vi "TLB Native Dynamic Events ver 0.13f.vi"() -> ()   [LabVIEW 2018]
uses:
  Labview Training Phase 2/Enum Controls/States for Action Engine.ctl
  TLB Type Definitions/State Type Definitions, for 0.26d versions and later.ctl
  TLB Type Definitions/Intruction Type Definitions.ctl
  TLB Type Definitions/Encoder cluster.ctl
  TLB Type Definitions/PING CLUSTER.ctl
  <vilib>/Studica/Studica Toolkit/NavX/NavX.lvlib
  <vilib>/Studica/Studica Toolkit/Background/DIO Channel.ctl
  Underlying VI's/NavX VI/navX type def.ctl
  <vilib>/myRIO/Instrument Drivers/Utilities/Utilities.lvlib
  <vilib>/Studica/Studica Toolkit/Background/I2C Channel.ctl
  TLB Type Definitions/Vision cluster.ctl
  <vilib>/NI_Real-Time Target Support.lvlib
  TLB Type Definitions/Stepper cluster.ctl
  Experimental VI's/Archived VI's/MOTOR CONTROL NO PID Type Def.ctl
  Underlying VI's/I2C Master VI/I2C MASTER Type Def.ctl
  Underlying VI's/I2C Master VI/I2C_MASTER_WRITE_NEW Type Def.ctl
  Underlying VI's/Webcam FGV Low level ver/State control.ctl
  <vilib>/userdefined/High Color/IMAQdx.ctl
  Underlying VI's/I2C Master VI/Arduino_Interfacing.ctl
  TLB Type Definitions/Yaw Cluster.ctl
  Experimental VI's/Archived VI's/MOTOR CONTROL NO PID AE DATA ENTRY MODE Type def.ctl
  Experimental VI's/Archived VI's/MOTOR CONTROL NO PID AE DIRECTIONS type def.ctl
  Underlying VI's/Elasped Timer/Control.ctl
  TLB Type Definitions/Time cluster.ctl
  TLB Type Definitions/Y Stepper cluster.ctl
  <vilib>/Utility/RT CPU Load.ctl
panel:
  out "Time up flag":bool
  out "Recognized object + Time up?":bool
  out "Speed & distance":T1
  out "Task selection":u8
  out "Object Center Coordinates":cluster{"x":sgl, "y":sgl}
  out "Object detection cluster":T2
  in  "Object recognition mode":enum16{"Ball", "Soap", "Gel", "Pipe", "None"}(ring)
  out "NavX Readings":T3
  out "Arduino Data":T4
  out "CPU loads":T5[](array[typedef]) {"ISR (%)" format="%#.2f"; "Idle (%)" format="%#.2f"; "Background (%)" format="%#.2f"; "Normal (%)" format="%#.2f"; "Above Normal (%)" format="%#.2f"; "High (%)" format="%#.2g"; "Timed Structures (%)" format="%#.2g"; "Time Critical (%)" format="%#.2g"; "Total (%)" format="%#.2g"}
  in  "Red LED":bool
  out "Detect?":bool
  out "TASK ENABLE":bool
  out "Rising Edge":bool
  in  "Green LED":bool
  out "Object detected?":bool
  out "I2C Error":errorcluster
  out "State Logic":T6=enum."Startup"
  out "elements":T7[](array[typedef])
  in  "STOP TASK":bool
  in  "OK Button":bool
  in  "STOP":bool
  out "error out":errorcluster
  out "Action Queue Items":i32
  out "State Logic Queue Items":i32
  out "Action Queues items":string[](array[string])=["Hardware reset", "Software reset", ""]
  out "Action State":string
  # "System Health Status Update"
  # "TLB FRAMEWORK STATUS"
  # "Test Programme written by Calvin Loke    Dated: 28 Aug 2019\nTest Programme revised by Dr Alex See   Dated 30 Aug 2019\n\nRevision date: 19/03/2020\nProgramme version:   TLB Native Dynamic Events ver 0.13f"
  # "VISION"
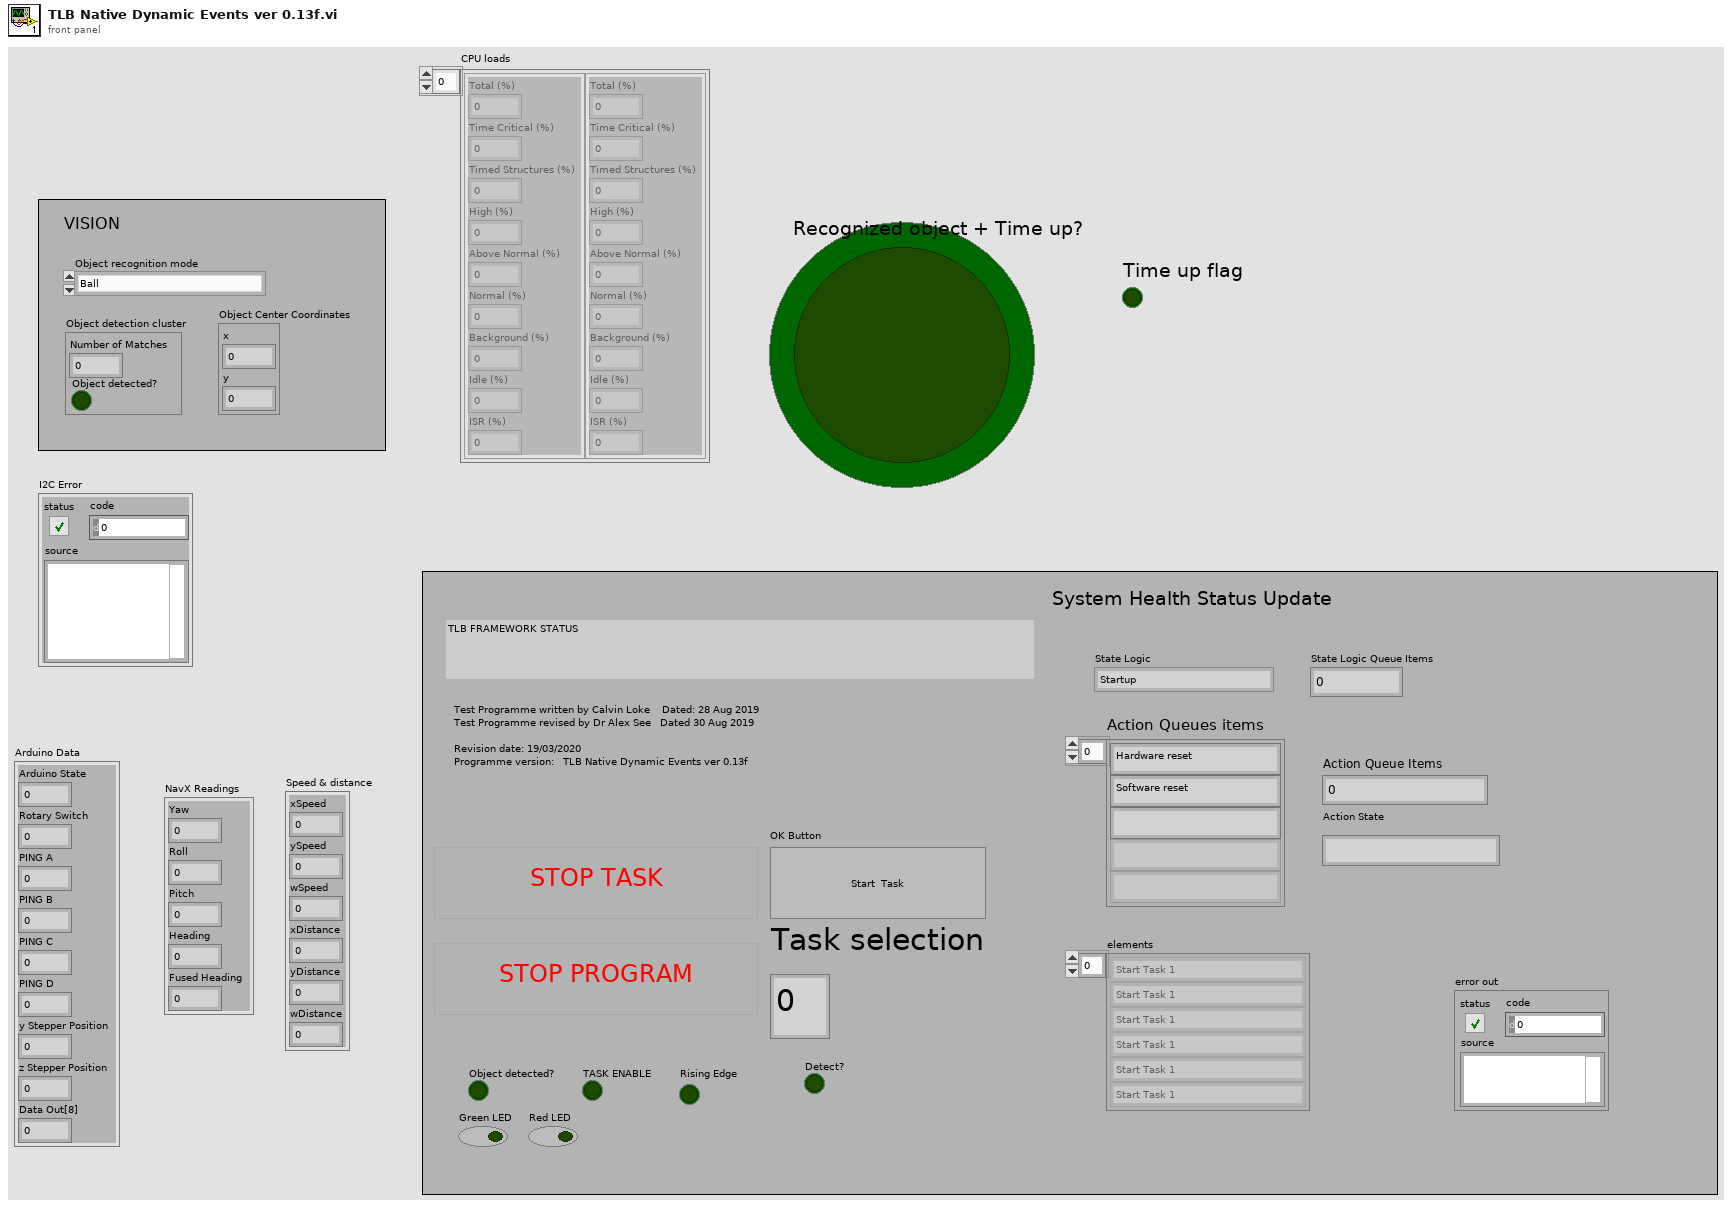
[diagram p1: front panel]
types:
  T1 = cluster{"xSpeed":dbl, "ySpeed":dbl, "wSpeed":dbl, "xDistance":dbl, "yDistance":dbl, "wDistance":dbl}
  T2 = cluster{"Number of Matches":i32, "Object detected?":bool}
  T3 = cluster{"Yaw":dbl, "Roll":dbl, "Pitch":dbl, "Heading":dbl, "Fused Heading":dbl}
  T4 = cluster{"Arduino State":u8, "Rotary Switch":u8, "PING A":u8, "PING B":u8, "PING C":u8, "PING D":u8, "y Stepper Position":u8, "z Stepper Position":u8, "Data Out[8]":u8}
  T5 = typedef "NI_Real-Time Target Support.lvlib/RT CPU Load.ctl" = cluster{"Total (%)":dbl, "Time Critical (%)":dbl, "Timed Structures (%)":dbl, "High (%)":dbl, "Above Normal (%)":dbl, "Normal (%)":dbl, "Background (%)":dbl, "Idle (%)":dbl, "ISR (%)":dbl}
  T6 = typedef "State Type Definitions.ctl" = enum16{"None", "Startup", "Move to Angle", "True Stop", "Idle", "Shutdown", "Task 1A", "Task 1B", "Task 2:Raise Arm", "Task 2:Sensor Mode", "Task 2:Reverse Mode", "Task 3", "Task 4_A", "Task 4_B", "Task 4_C", "Task 4_D", "Task 5A", "Task 5B", "Task 5C", "Task 5D", "Task 5E: POSITION ARM", "Task 5F: ARM GRAB HEIGHT", "Task 5G: CLOSE CLAW", "Task 5H: RAISE ARM", "Task 6_A", "Task 6_B", "Task 7", "Task 8A: RAISE ARM", "Task 8B: MOVE TO BOX", "Task 8C: CAM BURST", "Task 8D: PROCESS IMAGE", "Task 8E: ROBOT ADJUST", "Task 8F: CAM BURST 2", "Task 8G: PROCESS IMAGE 2", "Task 8H: ARM ADJUST", "Task 8I: ARM GRAB HEIGHT", "Task 8J: CLOSE CLAW", "Task 8K: RAISE MY SWORD", "Task 9A: Raise Arm", "Task 9B: Rotate to Angle", "Task 9C: Detect Box", "Task 9D: MOVE FORWARD", "Task 9E: MOVE LEFT", "Task 9F: SCAN IMAGE", "Task 9G: PROCESS COLOUR", "Task 9H: MOVE RIGHT", "Task 9I: SCAN IMAGE", "Task 9J: PROCESS COLOUR", "Task 9K: ROTATE 90 CW", "Task 9L: MOVE FORWARD", "Task 9M: MOVE RIGHT", "Task 9N: SCAN IMAGE", "Task 9O: PROCESS COLOUR", "Task 9P: MOVE RIGHT", "Task 9Q: SCAN IMAGE", "Task 9R: PROCESS COLOUR", "Task A1: Raise Arm", "Task A2: Rotate to Angle", "Task A3: Move Forward", "Task A4: Rotate CW 90"}
  T7 = typedef "Intruction Type Definitions.ctl" = enum16{"None", "Start Task 1", "Start Task 2", "Start Task 3", "Start Task 4", "Start Task 5", "Start Task 6", "Start Task 7", "Start Task 8 - BALL", "Start Task 8 - Gel", "Start Task 8 - Pipe", "Start Task 8 - Soap", "Start Task 9", "Start Task A", "Start Task B", "Exit"}
  T8 = typedef "Y Stepper cluster.ctl" = cluster{"yStepper desired":u8}
  T9 = typedef "Time cluster.ctl" = cluster{"Time up flag":bool, "SET TIME TO CHECK":dbl}
  T10 = typedef "Yaw Cluster.ctl" = cluster{"Yaw":dbl, "Compass":dbl}
  T11 = typedef "Stepper cluster.ctl" = cluster{"y Stepper Position":u8, "z Stepper Position":u8}
  T12 = typedef "DIO Channel.ctl" = enum16{"Not Connected", "A/DIO1", "A/DIO2", "A/DIO3", "A/DIO4", "A/DIO5", "A/DIO6", "A/DIO7", "A/DIO13", "B/DIO1", "B/DIO2", "B/DIO3", "B/DIO4", "B/DIO5", "B/DIO6", "B/DIO7", "B/DIO13", "C/DIO0", "C/DIO1", "C/DIO2", "C/DIO3", "C/DIO4", "C/DIO5", "C/DIO6", "C/DIO7"}
  T13 = typedef "Vision cluster.ctl" = cluster{"Recognized Object":bool, "Object X coordinate":dbl, "Object Y coordinate":dbl}
  T14 = typedef "PING CLUSTER.ctl" = cluster{"PING_A":u8, "PING_B":u8, "PING_C":u8, "PING_D":u8}
  T15 = typedef "Encoder cluster.ctl" = cluster{"xDistance":dbl, "yDistance":dbl, "wDistance":dbl}
  T16 = cluster{"DIO Channel":T12, "FPGA VI Reference Out":refnum<k20>}
  T17 = typedef "MOTOR CONTROL NO PID AE DATA ENTRY MODE Type def.ctl" = enum16{"Initialize", "Reset Encoders", "Write to motors", "Read from Encoders"}
  T18 = typedef "navX type def.ctl" = enum16{"Get i2C reference", "Read Values", "Zero Yaw"}
  T19 = typedef "Arduino_Interfacing.ctl" = enum16{"Initialize", "Write to Arduino", "Read From Arduino"}
  T20 = typedef "I2C Channel.ctl" = enum16{"Not Connected", "A", "B"}
  T21 = typedef "States for Action Engine.ctl" = enum16{"Initialize", "Write", "Read"}
  T22 = cluster{"I2C Ref Out":cluster{"I2C Channel":T20, "FPGA VI Reference Out":refnum<k20>}, "Connected":bool, "Slave Address (7-bit)":u8, "Registry":u8[]}
  T23 = typedef "IMAQ Image.ctl" = refnum<image>
  T24 = typedef "State Type Definitions.ctl" = enum16{"None", "Startup", "Move to Angle", "True Stop", "Idle", "Shutdown", "Task 1", "Task 2:Raise Arm", "Task 2:Sensor Mode", "Task 2:Reverse Mode", "Task 3", "Task 4_A", "Task 4_B", "Task 4_C", "Task 4_D", "Task 5A: ARM CAM HEIGHT", "Task 5B: MOVE TO BOX", "Task 5C: CAM BURST", "Task 5D: PROCESS IMAGE", "Task 5E: POSITION ARM", "Task 5F: ARM GRAB HEIGHT", "Task 5G: CLOSE CLAW", "Task 5H: RAISE ARM", "Task 6_A", "Task 6_B", "Task 7", "Task 8A: RAISE ARM", "Task 8B: MOVE TO BOX", "Task 8C: CAM BURST", "Task 8D: PROCESS IMAGE", "Task 8E: ROBOT ADJUST", "Task 8F: CAM BURST 2", "Task 8G: PROCESS IMAGE 2", "Task 8H: ARM ADJUST", "Task 8I: ARM GRAB HEIGHT", "Task 8J: CLOSE CLAW", "Task 8K: RAISE MY SWORD", "Task 9A: Raise Arm", "Task 9B: Rotate to Angle", "Task 9C: Detect Box", "Task 9D: MOVE FORWARD", "Task 9E: MOVE LEFT", "Task 9F: SCAN IMAGE", "Task 9G: PROCESS COLOUR", "Task 9H: MOVE RIGHT", "Task 9I: SCAN IMAGE", "Task 9J: PROCESS COLOUR", "Task 9K: ROTATE 90 CW", "Task 9L: MOVE FORWARD", "Task 9M: MOVE RIGHT", "Task 9N: SCAN IMAGE", "Task 9O: PROCESS COLOUR", "Task 9P: MOVE RIGHT", "Task 9Q: SCAN IMAGE", "Task 9R: PROCESS COLOUR"}
  T25 = typedef "State Type Definitions.ctl" = enum16{"None", "Startup", "Move to Angle", "True Stop", "Idle", "Shutdown", "Task 1", "Task 2", "Task 3", "Task 4_A", "Task 4_B", "Task 4_C", "Task 5_A", "Task 5 _B", "Task 5_C", "Task 5_C_Error", "Task 6_A", "Task 6_B", "Task 7", "Task 8", "Task 9", "Task A", "Task B"}
  T26 = typedef "MOTOR CONTROL NO PID AE DIRECTIONS type def.ctl" = enum16{"y-axis movement", "x-axis movement", "Rotate", "Stop"}
  T27 = typedef "Control.ctl" = enum16{"Start", "Pause", "Initialize"}
  T28 = typedef "I2C_MASTER_WRITE_NEW Type Def.ctl" = enum16{"Ultrasonic sensors", "Stepper origin", "zStepper 13.3k", "zStepper 13k", "zStepper 12k", "zStepper 11k", "zStepper 10k", "zStepper 9k", "zStepper 8k", "zStepper 7k", "zStepper 6k", "zStepper 5k", "zStepper 4k", "zStepper 3k", "zStepper 2k", "zStepper 1k", "zStepper 900", "zStepper 800", "zStepper 700", "zStepper 600", "zStepper 500", "zStepper 400", "zStepper 300", "zStepper 200", "zStepper 100", "zStepper 0", "yStepper control", "Open Claw", "Close Claw", "Soft Reset"}
  T29 = typedef "State control.ctl" = enum16{"Initialise", "Start camera", "Continuous Acquisition ", "Stop camera", "Dispose all"}
  T30 = typedef "IMAQdx.ctl" = refnum<k21>
  T31 = typedef "MOTOR CONTROL NO PID Type Def.ctl" = enum16{"Init", "Front Back", "Left Right", "Rotate", "Stop", "Latch"}
  T32 = typedef "I2C MASTER Type Def.ctl" = enum16{"Last State", "Mode 0", "Mode 1", "Mode 2", "Mode 3", "Mode 4", "Mode 5", "Mode 6", "Mode 7", "Mode 8", "Mode 9", "Mode 10"}
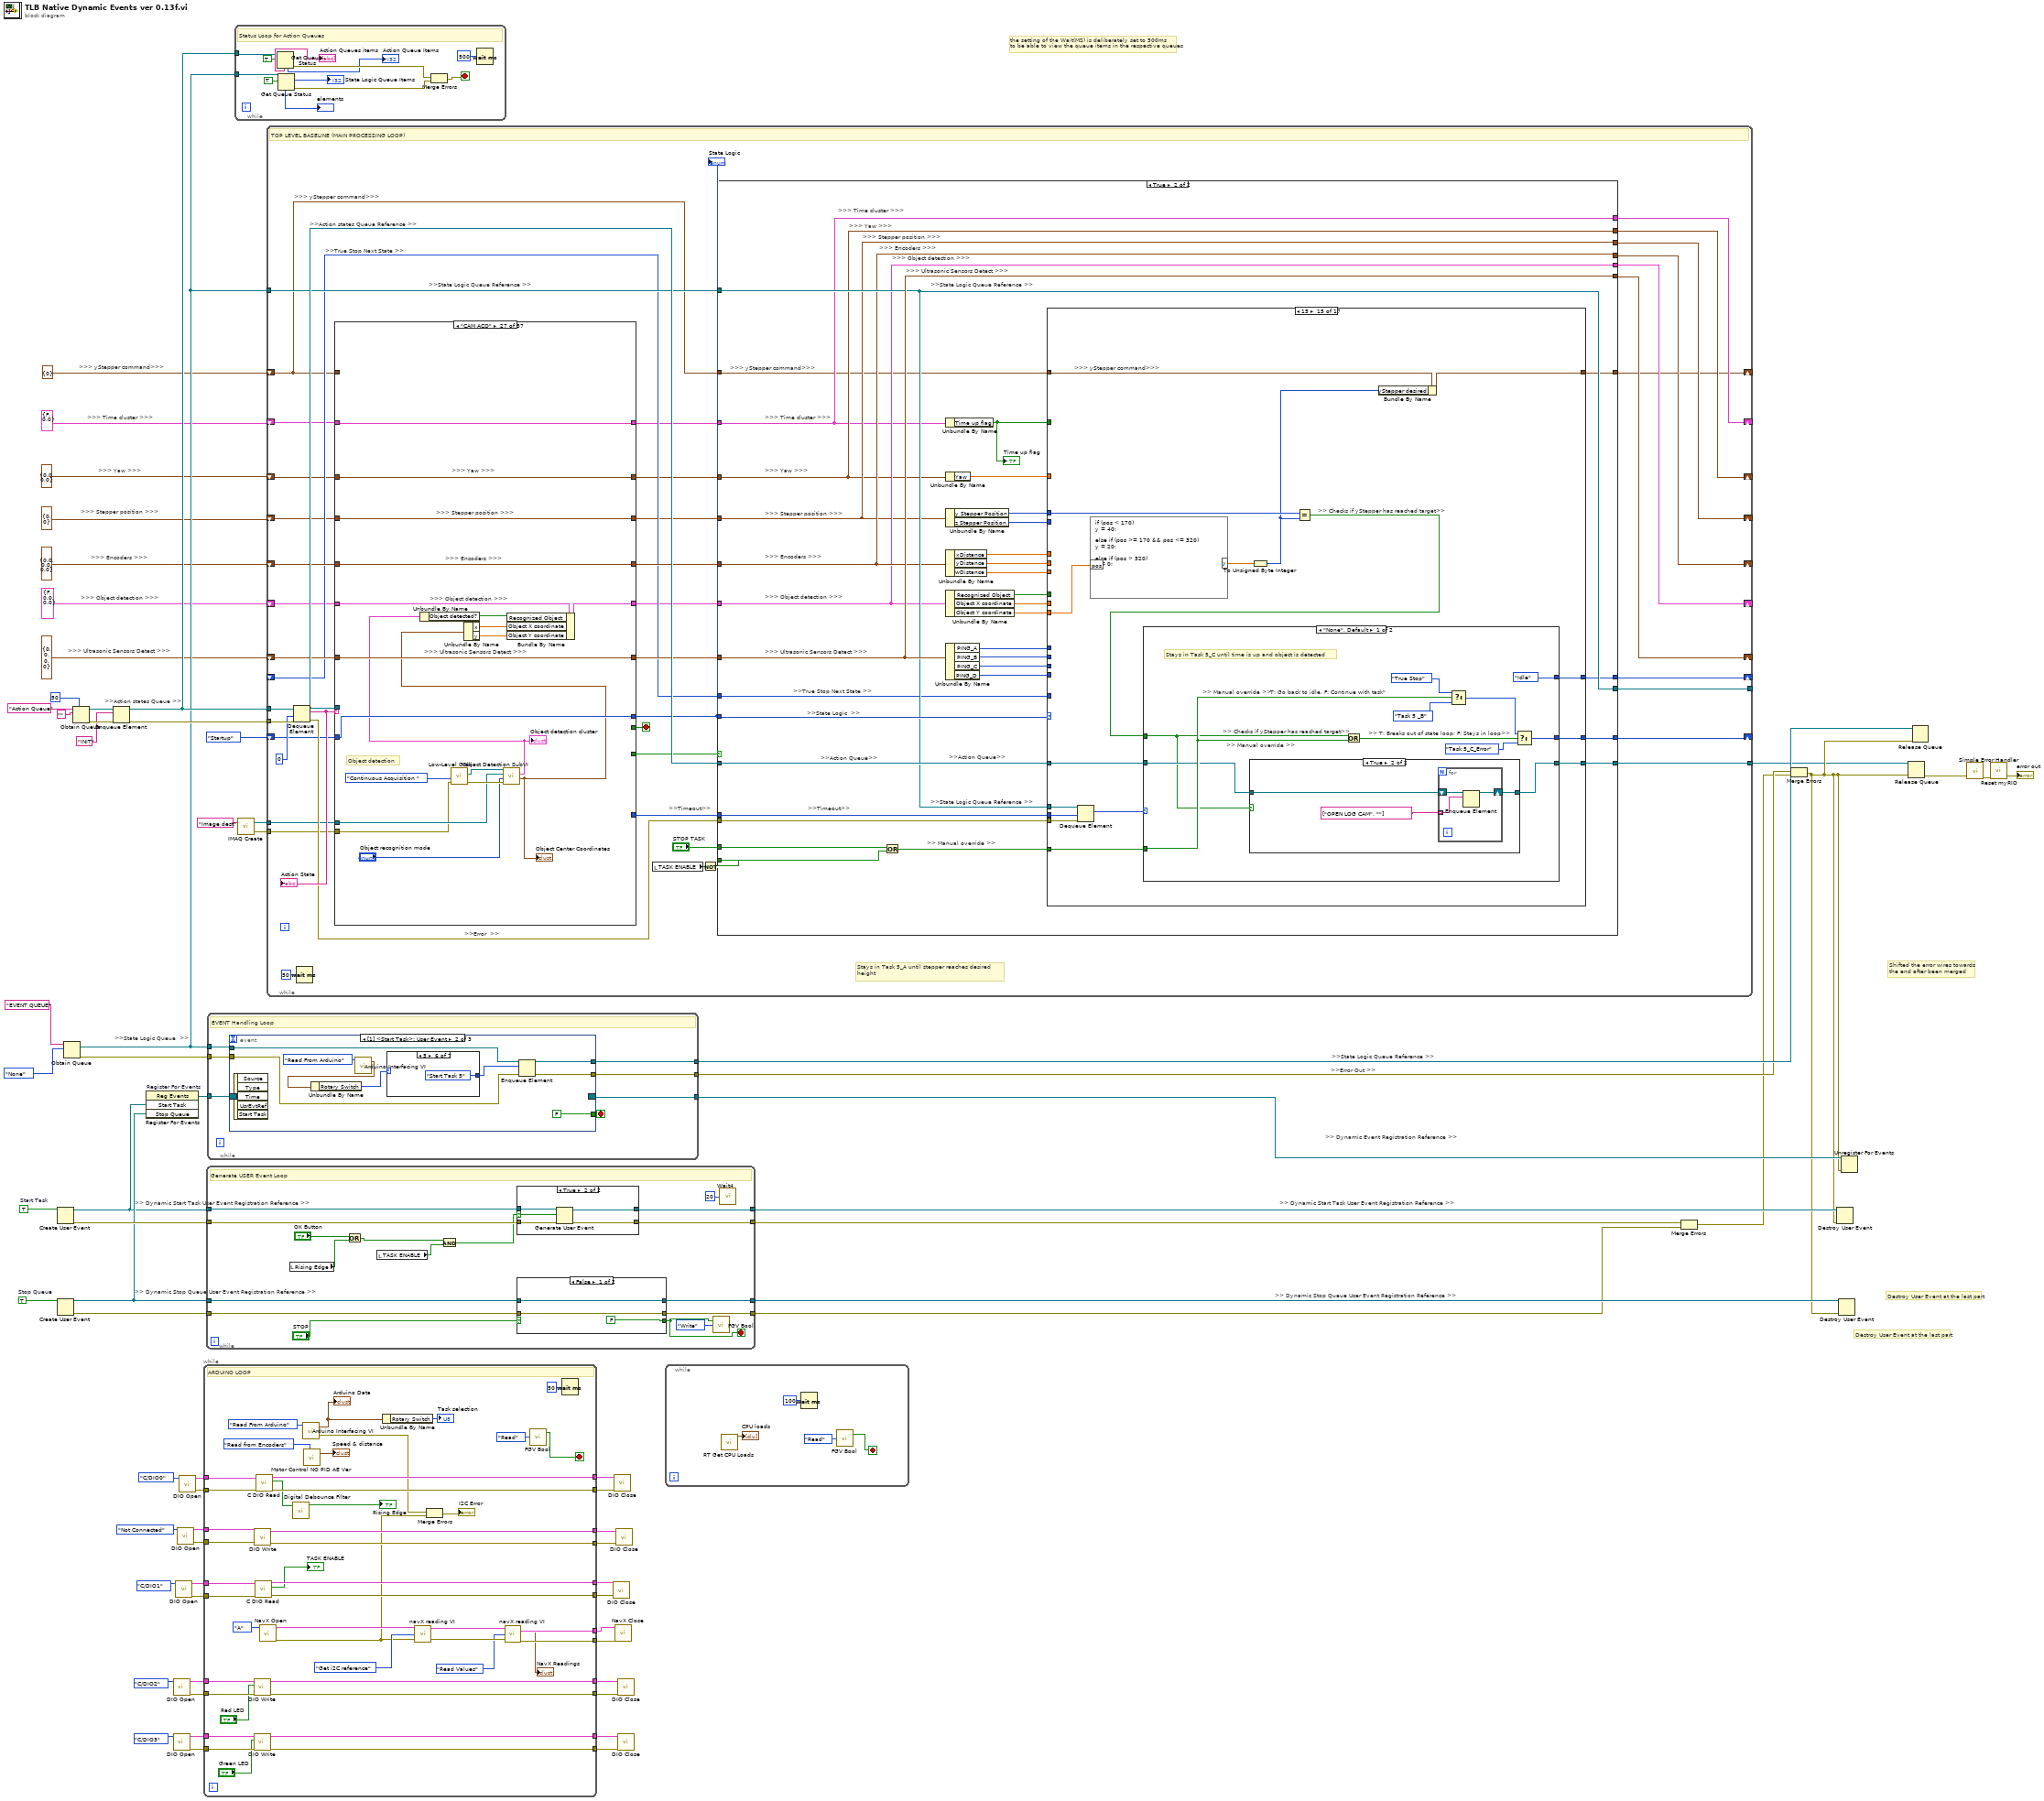
[diagram p0: block diagram]
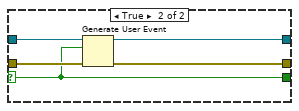
[diagram p2: hidden frame]
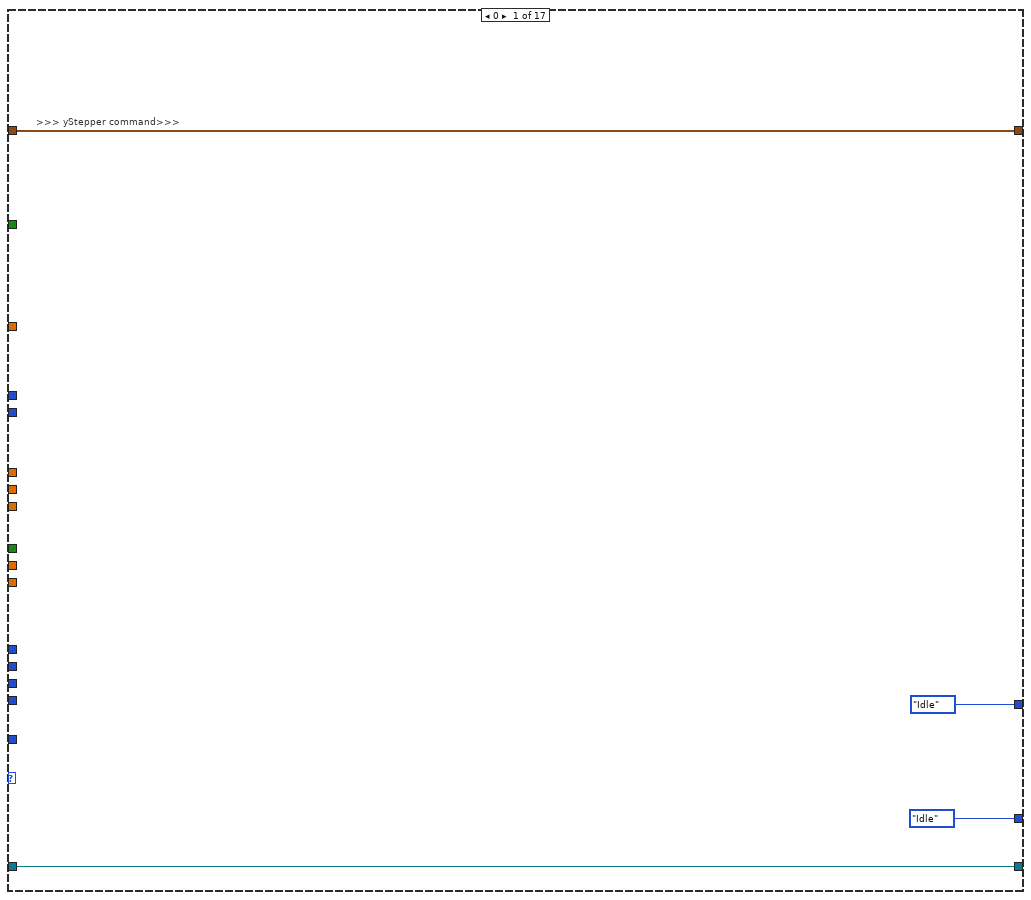
[diagram p5: hidden frame]
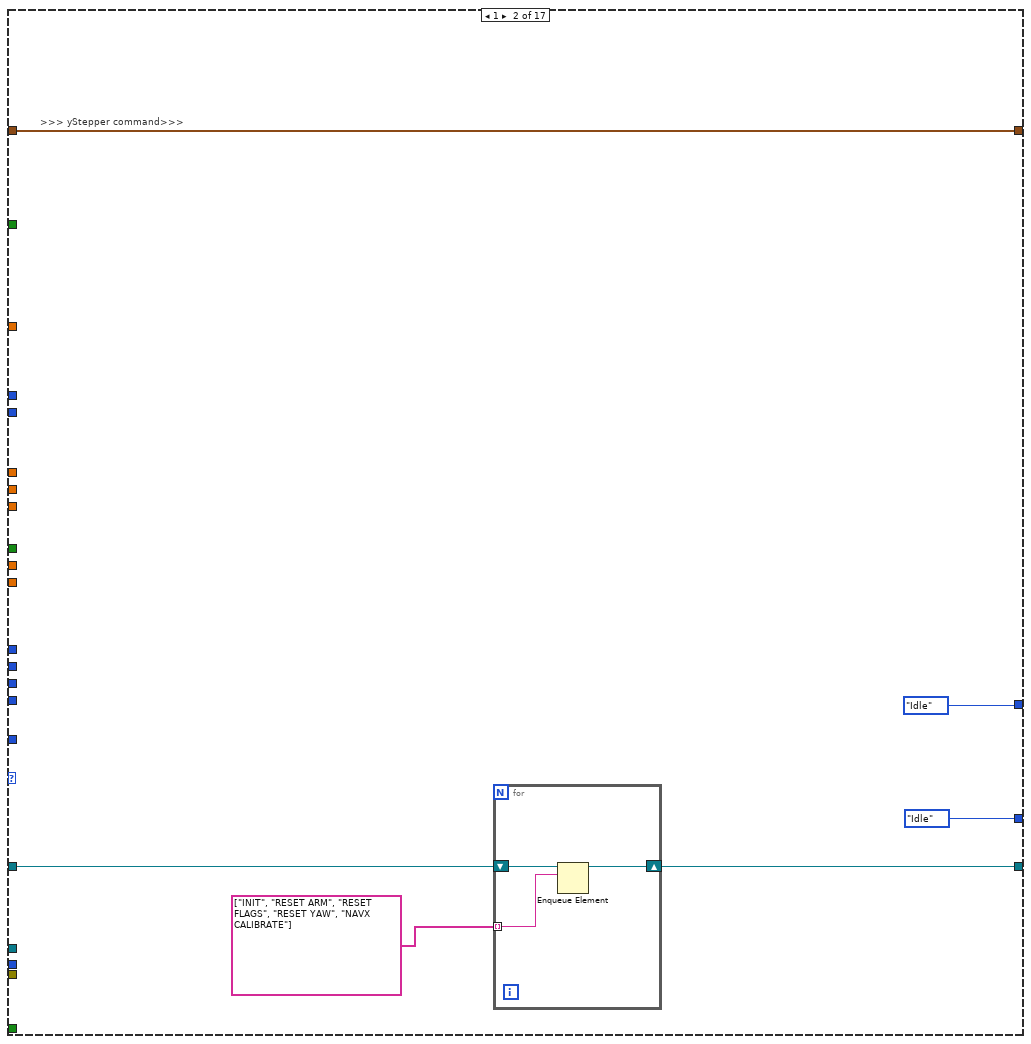
[diagram p6: hidden frame]
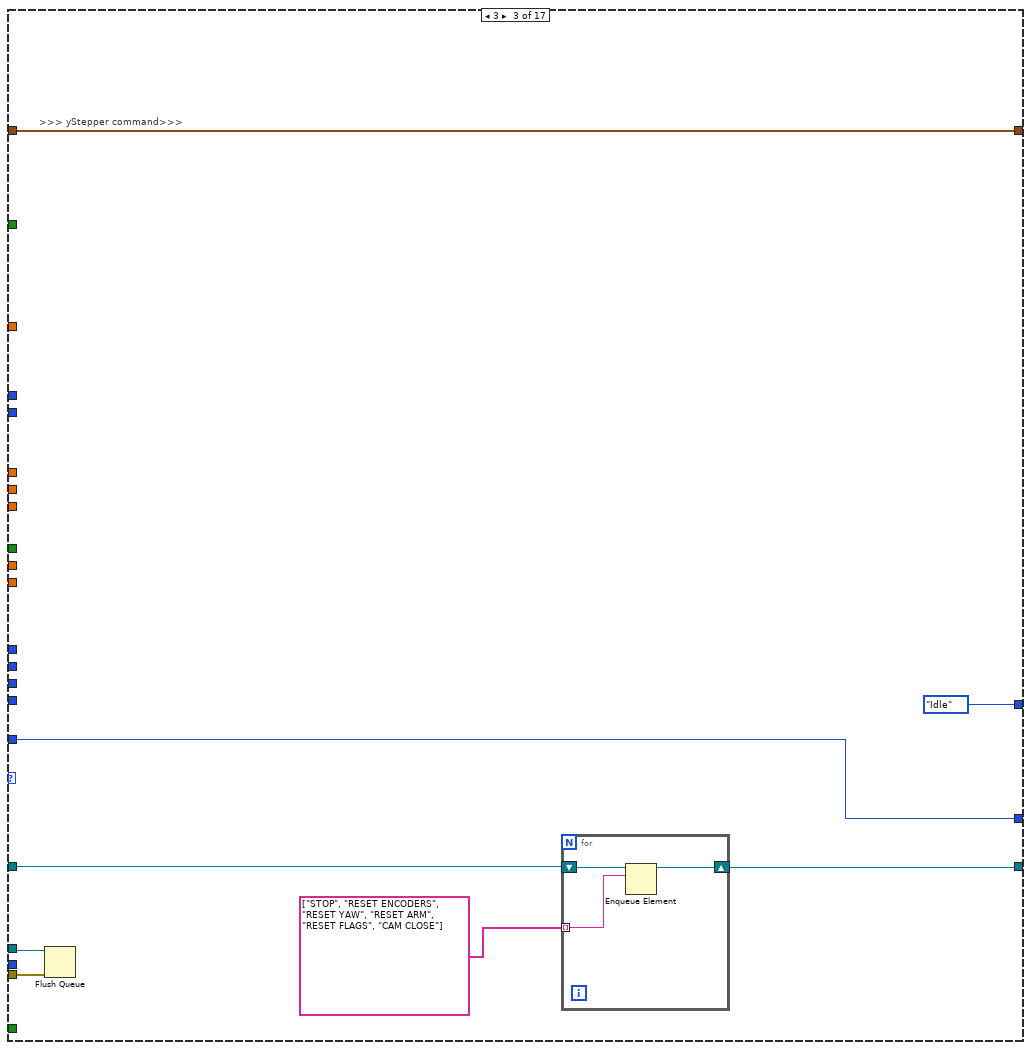
[diagram p7: hidden frame]
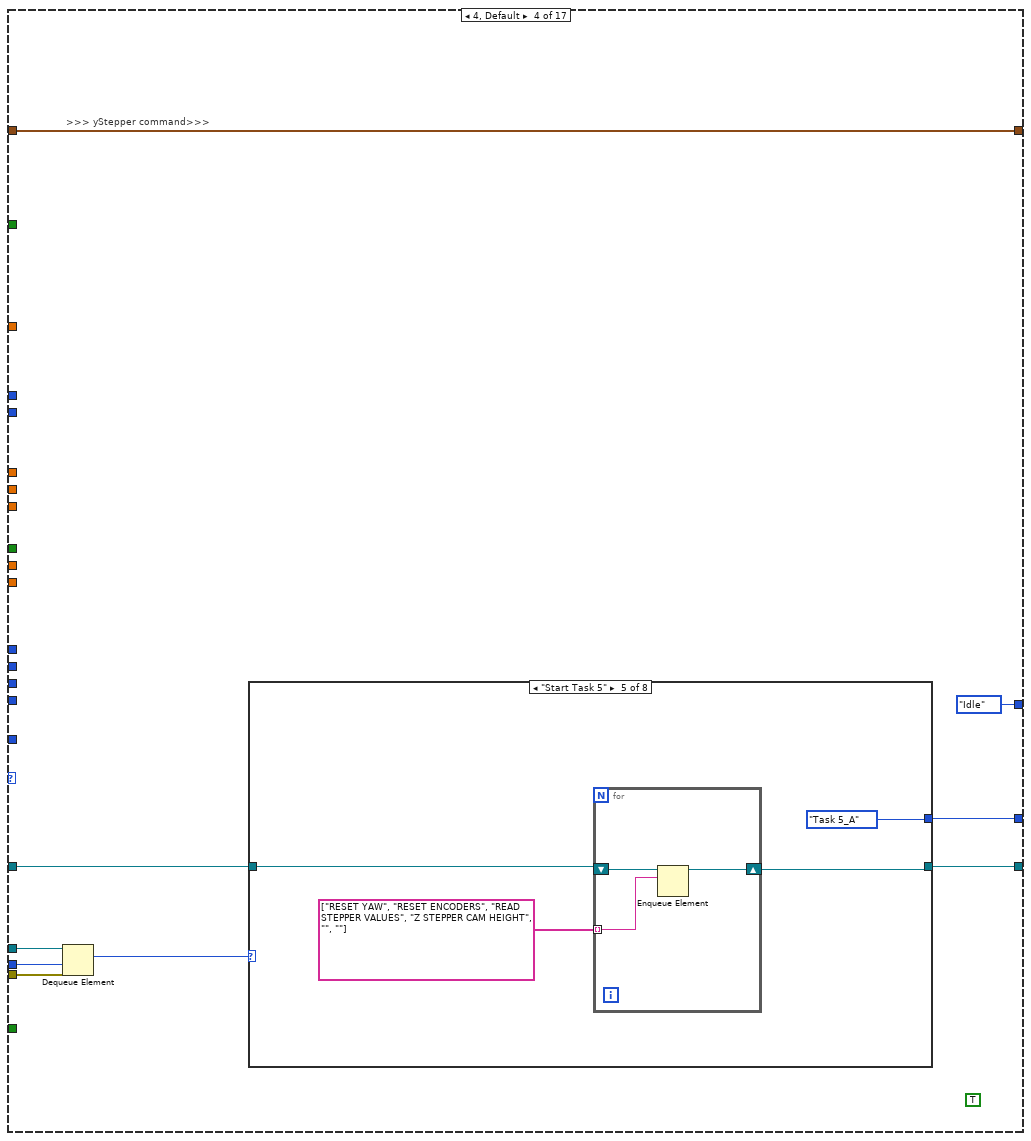
[diagram p8: hidden frame]
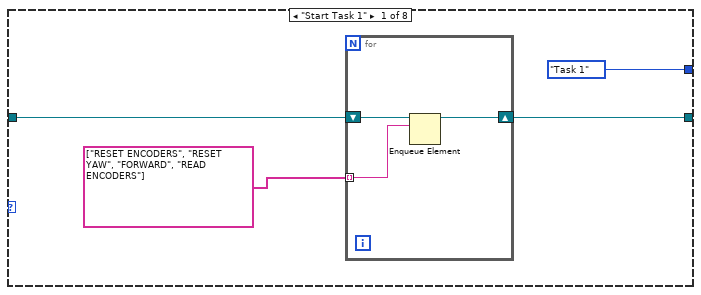
[diagram p9: hidden frame]
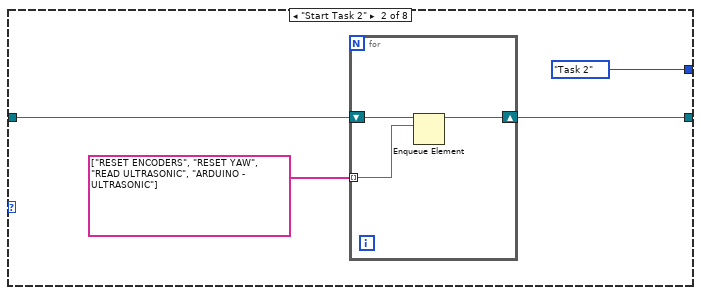
[diagram p10: hidden frame]
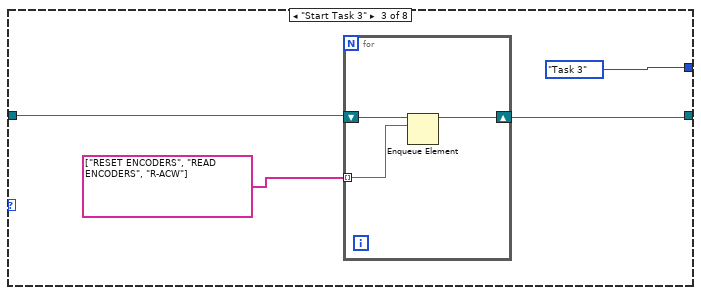
[diagram p11: hidden frame]
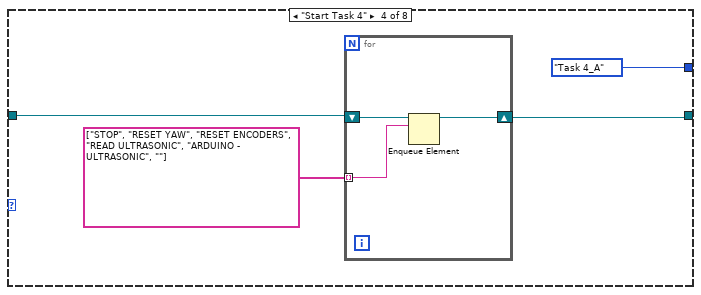
[diagram p12: hidden frame]
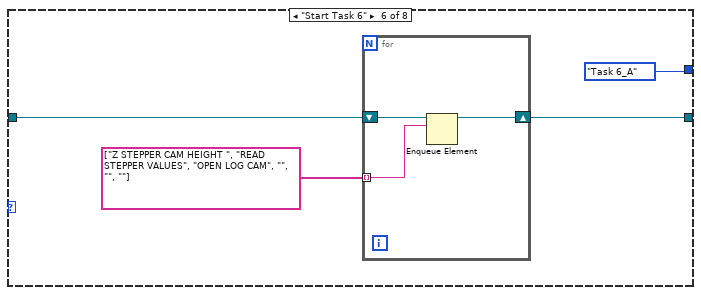
[diagram p13: hidden frame]
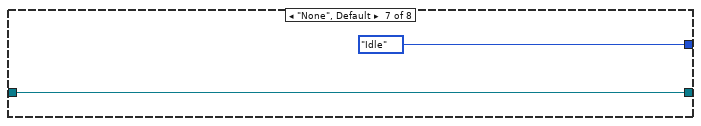
[diagram p14: hidden frame]
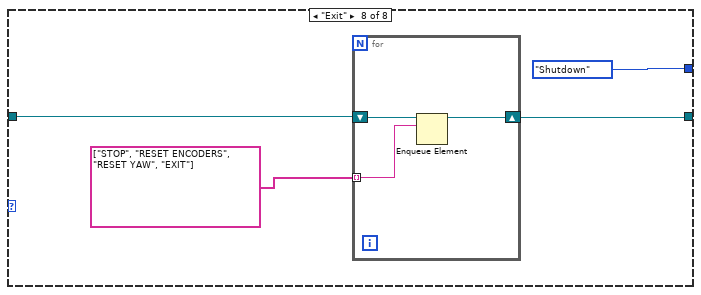
[diagram p15: hidden frame]
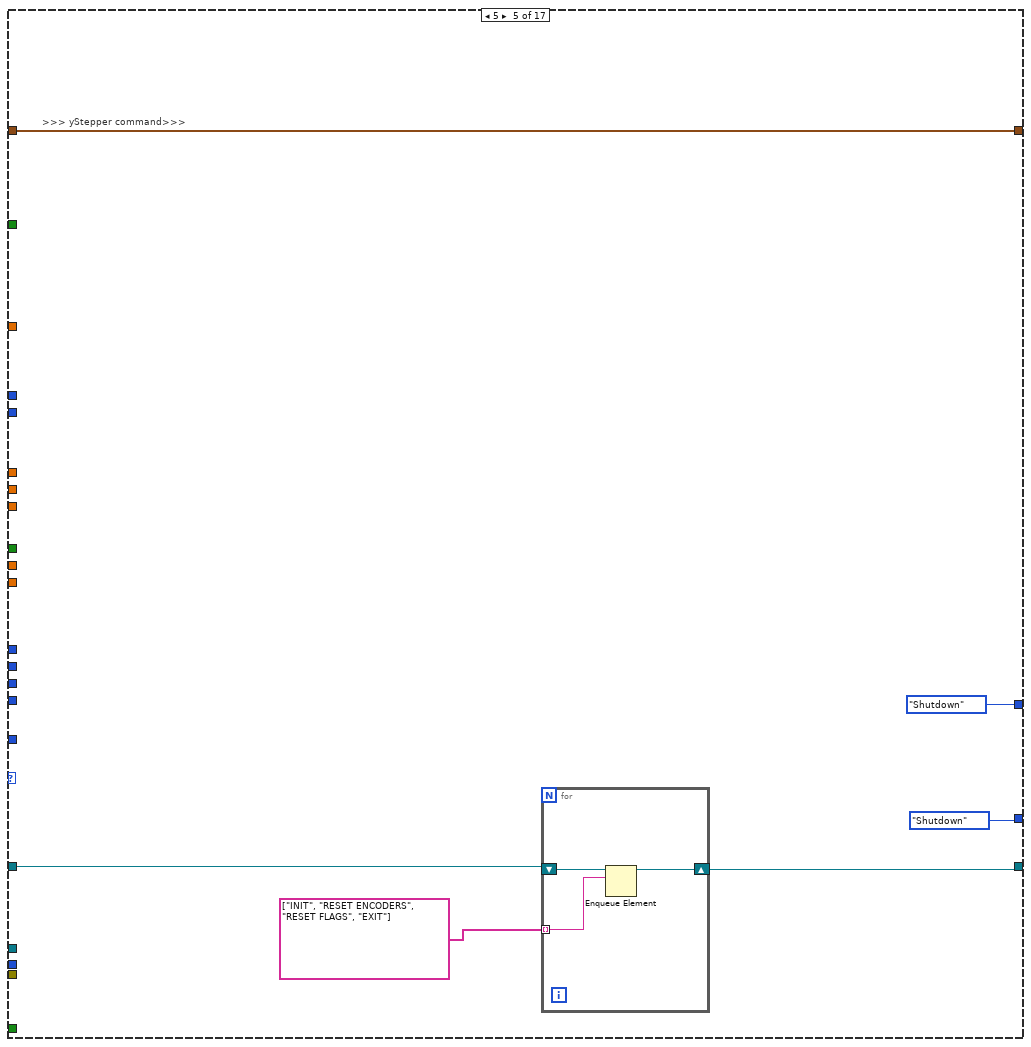
[diagram p16: hidden frame]
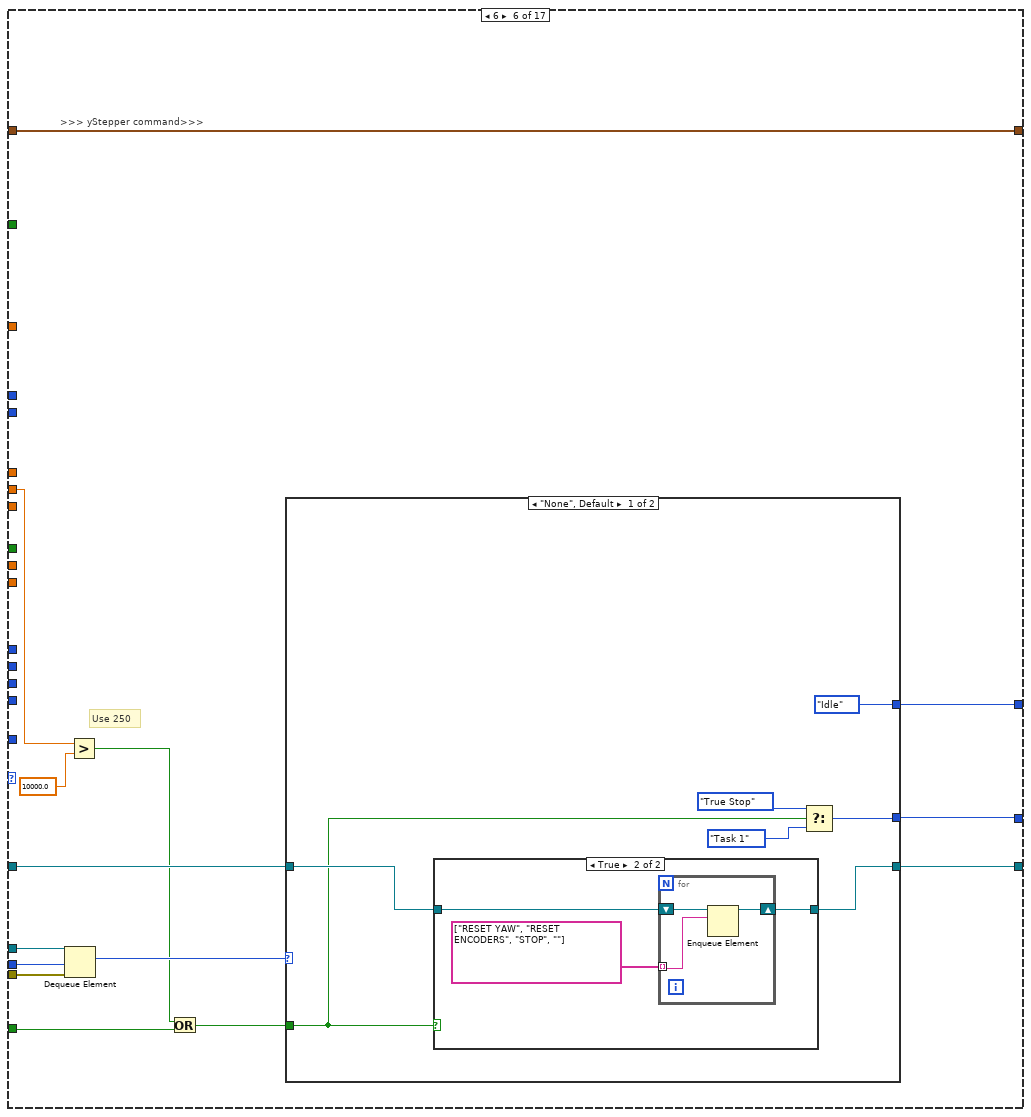
[diagram p17: hidden frame]
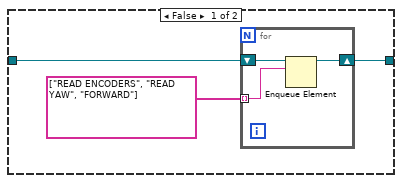
[diagram p18: hidden frame]
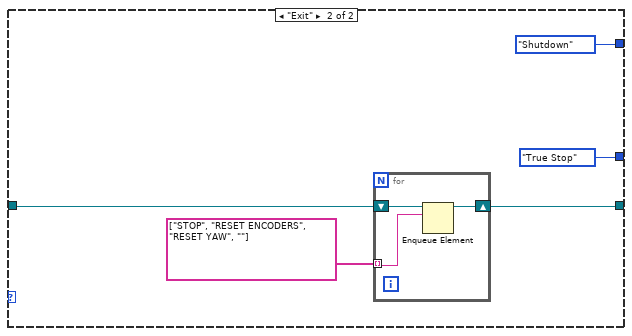
[diagram p19: hidden frame]
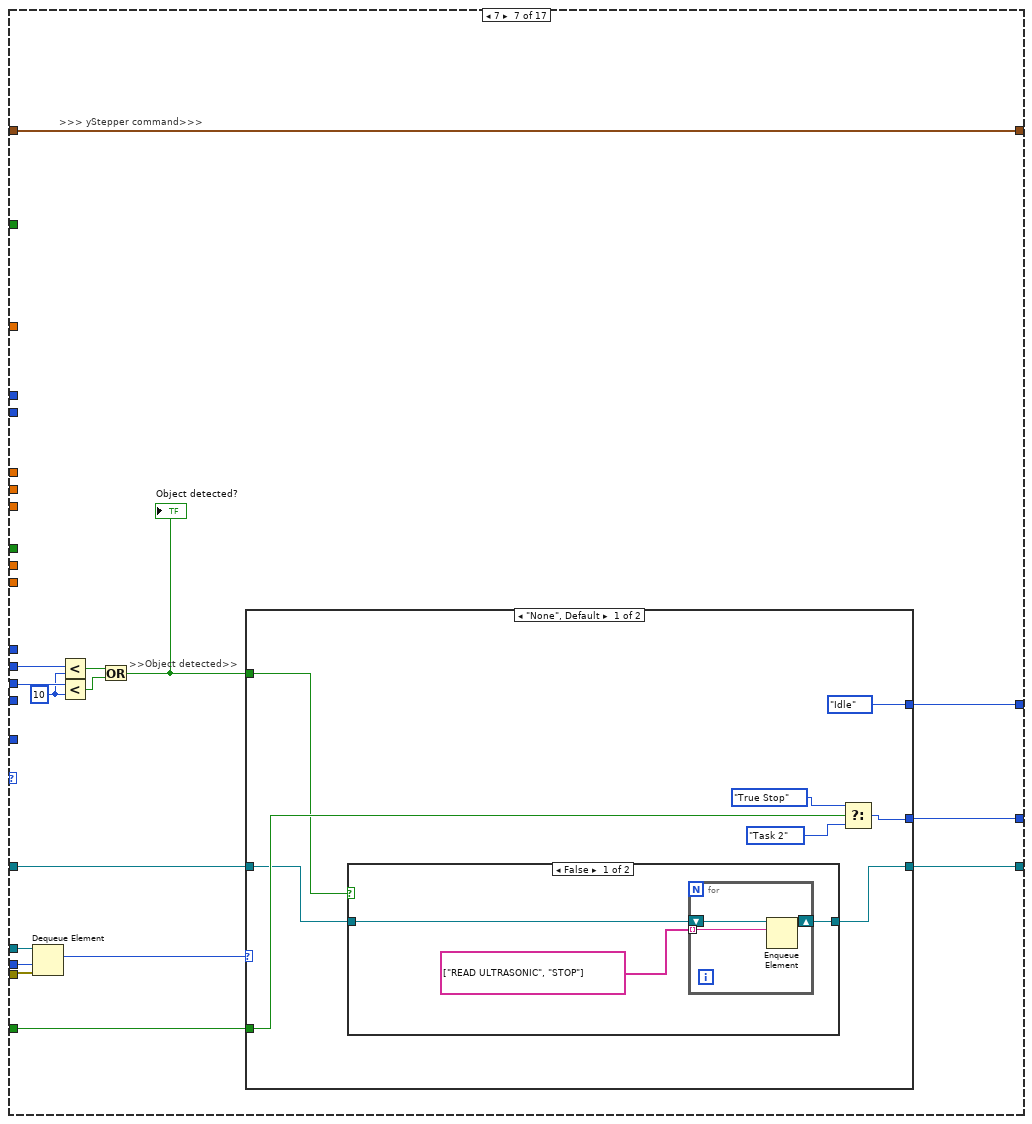
[diagram p20: hidden frame]
diagram:
  w70 = TRUE  # Stop Queue
  w69 = TRUE  # Start Task
  # ">>> yStepper command>>>"
  # ">>> Time cluster >>>"
  # ">>> Yaw >>>"
  # ">>> Stepper position >>>"
  # ">>> Encoders >>>"
  # ">>> Object detection >>>"
  # ">>> Ultrasonic Sensors Detect >>>"
  # "the setting of the Wait(MS) is deliberately set to 500ms\nto be able to view the queue items in the respective queues"
  # ">>Error Out >>"
  # ">> Dynamic Stop Queue User Event Registration Reference >>"
  # ">> Dynamic Start Task User Event Registration Reference >>"
  # ">> Dynamic Stop Queue User Event Registration Reference >>"
  # ">> Dynamic Start Task User Event Registration Reference >>"
  # ">> Dynamic Event Registration Reference >>"
  # ">>Action states Queue >>"
  # ">>State Logic Queue  >>"
  # ">>State Logic Queue Reference >>"
  # "Destroy User Event at the last part"
  # "Destroy User Event at the last part"
  # "Shifted the error wires towards\nthe end after been merged"
  n1 = Create User Event(user event datatype=w69) -> (user event=w61:refnum<user-event>, error out=w66:errorcluster)  [unwired: 1 in]
  n2 = Create User Event(user event datatype=w70) -> (user event=w62:refnum<user-event>, error out=w65:errorcluster)  [unwired: 1 in]
  n3 = Obtain Queue(name (unnamed)="EVENT QUEUE", element data type=Intruction_Type_Definitions."None" ("Enum")) -> (queue out=w47:refnum<queue>, error out=w53:errorcluster)  [unwired: 3 in, 1 out]
  n4 = Obtain Queue(max queue size (-1, unlimited)=50, name (unnamed)="Action Queue", element data type="") -> (queue out=w56:refnum<queue>, error out=w52:errorcluster)  [unwired: 2 in, 1 out]
  n5 = Enqueue Element(queue=w56, element="INIT", error in (no error)=w52) -> (queue out=w48:refnum<queue>, error out=w51:errorcluster)  [unwired: 1 in, 1 out]
  n6 = register-events "Register For Events"(w61, w62) -> (reference out=w60:refnum<event-registration>)  [unwired: 2 in, 1 out]
  n7 = call <vilib>:"DIO Open.vi"("DIO Channel"=DIO_Channel."C/DIO2") -> ("error out"=w14:errorcluster, "DIO Info Out"=w15:T16)  [unwired: 9 in]
  n8 = call <vilib>:"DIO Open.vi"("DIO Channel"=DIO_Channel."C/DIO3") -> ("error out"=w9:errorcluster, "DIO Info Out"=w10:T16)  [unwired: 9 in]
  n9 = call <vilib>:"DIO Open.vi"("DIO Channel"=DIO_Channel."C/DIO1") -> ("error out"=w25:errorcluster, "DIO Info Out"=w26:T16)  [unwired: 9 in]
  n10 = call <vilib>:"DIO Open.vi"("DIO Channel"=DIO_Channel."Not Connected") -> ("error out"=w30:errorcluster, "DIO Info Out"=w32:T16)  [unwired: 9 in]
  n11 = call <vilib>:"DIO Open.vi"("DIO Channel"=DIO_Channel."C/DIO0") -> ("error out"=w35:errorcluster, "DIO Info Out"=w38:T16)  [unwired: 9 in]
  n12 = while {
    tunnel: w38 -> [w112]
    tunnel: [w111] -> w36
    tunnel: w35 -> [w110]
    tunnel: [w109] -> w34
    tunnel: w32 -> [w105]
    tunnel: [w104] -> w31
    tunnel: w30 -> [w103]
    tunnel: [w102] -> w29
    tunnel: [w101] -> w27
    tunnel: w26 -> [w100]
    tunnel: w25 -> [w99]
    tunnel: [w98] -> w24
    tunnel: w15 -> [w92]
    tunnel: w14 -> [w91]
    tunnel: [w90] -> w13
    tunnel: [w89] -> w12
    tunnel: w10 -> [w87]
    tunnel: w9 -> [w86]
    tunnel: [w85] -> w8
    tunnel: [w84] -> w7
    tunnel: [w78] -> w4
    tunnel: [w77] -> w5
    stop <- w114 stop-if-true
    # "ARDUINO LOOP"
    n13 = call <vilib>:"DIO Write.vi"("error in (no error)"=w91, "Input"="Red LED", "DIO Info In"=w92) -> ("error out"=w89:errorcluster, "DIO Info Out"=w90:T16)  [unwired: 7 in]
    n14 = call <vilib>:"DIO Write.vi"("error in (no error)"=w86, "Input"="Green LED", "DIO Info In"=w87) -> ("error out"=w84:errorcluster, "DIO Info Out"=w85:T16)  [unwired: 7 in]
    n15 = call <vilib>:"DIO Write.vi"("error in (no error)"=w103, "DIO Info In"=w105) -> ("error out"=w102:errorcluster, "DIO Info Out"=w104:T16)  [unwired: 8 in]
    n16 = call <vilib>:"C DIO Read.vi"("error in (no error)"=w99, "DIO Info In in"=w100) -> ("error out"=w98:errorcluster, "IN"=→"TASK ENABLE":bool, "DIO Info In out"=w101:T16)  [unwired: 7 in]
    n17 = call <vilib>:"C DIO Read.vi"("error in (no error)"=w110, "DIO Info In in"=w112) -> ("error out"=w109:errorcluster, "IN"=w107:bool, "DIO Info In out"=w111:T16)  [unwired: 7 in]
    n18 = call <vilib>:"NavX Open.vi"("I2C Channel"=I2C_Channel."A") -> ("error out"=w94:errorcluster, "NavX Info"=w96:T22)  [unwired: 9 in]
    n19 = call "Digital Debounce Filter.vi"("Boolean input"=w107) -> ("Rising Edge"=→"Rising Edge":bool)  [unwired: 1 in, 2 out]
    n20 = call "Arduino Interfacing VI.vi"("AE Mode"=Arduino_Interfacing."Read From Arduino") -> ("error out"=w81:errorcluster, "Arduino Data"=w74:T4)  [unwired: 3 in]
    "Arduino Data" <- w74
    n21 = call "Motor Control NO PID AE Ver.vi"("AE Mode"=MOTOR_CONTROL_NO_PID_AE_DATA_ENTRY_MODE_Type_def."Read from Encoders") -> ("Speed & distance"=→"Speed & distance":T1)  [unwired: 4 in, 1 out]
    n22 = Unbundle By Name(w74) -> ("Rotary Switch"=→"Task selection":u8)
    n23 = call "navX reading VI.vi"("NavX Info In"=w96, "Mode"=navX_type_def."Get i2C reference", "error in (no error)"=w94) -> ("NavX Info Out"=w80:T22, "Error Out"=w79:errorcluster)  [unwired: 2 out]
    n24 = Merge Errors(w81, w94) -> (→"I2C Error":errorcluster)
    n25 = call "navX reading VI.vi"("NavX Info In"=w80, "Mode"=navX_type_def."Read Values", "error in (no error)"=w79) -> ("NavX Info Out"=w78:T22, "NavX Readings"=→"NavX Readings":T3, "Error Out"=w77:errorcluster)  [unwired: 1 out]
    n26 = call "FGV Bool.vi"("Init/Read/Write State"=States_for_Action_Engine."Read") -> ("Output node"=w114:bool)  [unwired: 2 in, 1 out]
    n27 = Wait (ms)(milliseconds to wait=u32 50) -> ()  [unwired: 1 out]
  }
  n28 = while {
    tunnel: w61 -> [w132]
    tunnel: w62 -> [w131]
    tunnel: [w130] -> w68
    tunnel: [w129] -> w67
    tunnel: w66 -> [w128]
    tunnel: [w127] -> w64
    tunnel: w65 -> [w126]
    tunnel: [w125] -> w63
    stop <- w123 stop-if-true
    # "Generate USER Event Loop"
    n29 = local read "Rising Edge"() -> (w119:bool)
    n30 = Or(x="OK Button", y=w119) -> (x .or. y?=w118:bool)
    n31 = local read "TASK ENABLE"() -> (w117:bool)
    n32 = And(x=w118, y=w117) -> (x .and. y?=w116:bool)
    n33 = case shown="True" w116 {
      selector: w116 -> [_ w143]
      tunnel: w132 -> [w142 w147]
      tunnel: [w142 w146] -> w129
      tunnel: w128 -> [w141 w145]
      tunnel: [w141 w144] -> w127
      frame False {
      }
      frame True {
        n34 = Generate User Event(user event=w147, event data cluster=w143, error in=w145) -> (user event out=w146:refnum<user-event>, error out=w144:errorcluster)  [unwired: 1 in]
      }
    }
    n35 = case shown="False" "STOP" {
      selector: "STOP" -> [_ w136]
      tunnel: w131 -> [w135 w140]
      tunnel: [w135 w139] -> w130
      tunnel: w126 -> [w134 w138]
      tunnel: [w134 w137] -> w125
      tunnel: [FALSE w136] -> w123
      frame False {
      }
      frame True {
        n36 = Generate User Event(user event=w140, event data cluster=w136, error in=w138) -> (user event out=w139:refnum<user-event>, error out=w137:errorcluster)  [unwired: 1 in]
      }
    }
    n37 = call "FGV Bool.vi"("Init/Read/Write State"=States_for_Action_Engine."Write", "Input Node"=w123) -> ()  [unwired: 1 in, 2 out]
    n38 = call "Wait4"("Count(uSec)"=u32 20) -> ()  [unwired: 1 out]
  }
  n39 = while {
    tunnel: w60 -> [w154]
    tunnel: [w153] -> w59
    tunnel: w47 -> [w151]
    tunnel: [w150] -> w58
    tunnel: w53 -> [w149]
    tunnel: [w148] -> w50
    stop <- w152 stop-if-true
    # "EVENT Handling Loop"
    n40 = event shown="[1] <Start Task>: User Event" {
      selector: w154 -> [_ _ _]
      dyn-events: [_ _ _] -> w153
      timeout: _ -> [_ _ _]
      tunnel: [FALSE FALSE w182] -> w152
      tunnel: w151 -> [w159 w168 w180]
      tunnel: [w158 w167 w181] -> w150
      tunnel: w149 -> [w157 w166 w179]
      tunnel: [w156 w165 w178] -> w148
      event Timeout {
        n41 = event-data() -> ()  [unwired: 1 in, 3 out]
        n42 = Enqueue Element(queue=w159, element=Intruction_Type_Definitions."None" ("Enum"), error in (no error)=w157) -> (queue out=w158:refnum<queue>, error out=w156:errorcluster)  [unwired: 1 in, 1 out]
      }
      event User Event {
        n43 = event-data() -> ()  [unwired: 1 in, 5 out]
        n44 = call "Arduino Interfacing VI.vi"("AE Mode"=Arduino_Interfacing."Read From Arduino") -> ("Arduino Data"=w162:T4)  [unwired: 3 in, 1 out]
        n45 = Unbundle By Name(w162) -> ("Rotary Switch"=w161:u8)
        n46 = case shown="5" w161 {
          tunnel: [Intruction_Type_Definitions."None" ("Enum") Intruction_Type_Definitions."Start Task 1" ("Enum") Intruction_Type_Definitions."Start Task 2" ("Enum") Intruction_Type_Definitions."Start Task 3" ("Enum") Intruction_Type_Definitions."Start Task 4" ("Enum") Intruction_Type_Definitions."Start Task 5" ("Enum") Intruction_Type_Definitions."Start Task 6" ("Enum")] -> w164
          frame 0, Default {
          }
          frame 1 {
          }
          frame 2 {
          }
          frame 3 {
          }
          frame 4 {
          }
          frame 5 {
          }
          frame 6 {
          }
        }
        n47 = Enqueue Element(queue=w168, element=w164, error in (no error)=w166) -> (queue out=w167:refnum<queue>, error out=w165:errorcluster)  [unwired: 1 in, 1 out]
      }
      event User Event {
        n48 = event-data() -> ("Stop Queue"=w182:bool)  [unwired: 1 in, 4 out]
        n49 = Enqueue Element At Opposite End(queue=w180, element=Intruction_Type_Definitions."Exit" ("Enum"), error in (no error)=w179) -> (queue out=w181:refnum<queue>, error out=w178:errorcluster)  [unwired: 1 in, 1 out]
      }
    }
  }
  n50 = while {
    tunnel: w48 -> [w192]
    tunnel: w47 -> [w189]
    stop <- w186 stop-if-true
    # "Status Loop for Action Queues"
    n51 = Get Queue Status(queue=w192, return elements? (F)=TRUE) -> (error out=w188:errorcluster, # elements in queue=→"Action Queue Items":i32, elements=→"Action Queues items":string[])  [unwired: 1 in, 5 out]
    n52 = Get Queue Status(queue=w189, return elements? (F)=TRUE) -> (# pending remove=→"State Logic Queue Items":i32, error out=w187:errorcluster, elements=→"elements":T7[])  [unwired: 1 in, 5 out]
    n53 = Merge Errors(w188, w187) -> (w186:errorcluster)
    n54 = Wait (ms)(milliseconds to wait=u32 500) -> ()  [unwired: 1 out]
  }
  n55 = call "IMAQ Create"("Image Name"="Image dest") -> ("New Image"=w19:T23, "error out"=w18:errorcluster)  [unwired: 4 in]
  n56 = while {
    tunnel: w47 -> [w225]
    tunnel: w48 -> [w237]
    tunnel: w51 -> [w235]
    tunnel: [w234] -> _
    tunnel: [w233] -> w41
    shift-right: [w226] -> _
    shift-left: T14 {"PING_A"=0, "PING_B"=0, "PING_C"=0, "PING_D"=0} -> [w228]
    shift-right: [w219] -> _
    shift-left: State_Type_Definitions."Startup" ("Enum") -> [w222]
    shift-right: [w215] -> _
    shift-left: T15 {"xDistance"=0.0, "yDistance"=0.0, "wDistance"=0.0} -> [w217]
    shift-right: [w212] -> _
    shift-left: _ -> [w211]
    tunnel: w19 -> [w210]
    tunnel: w18 -> [w209]
    shift-right: [w206] -> _
    shift-left: T13 {"Recognized Object"=FALSE, "Object X coordinate"=0.0, "Object Y coordinate"=0.0} -> [w208]
    shift-right: [w203] -> _
    shift-left: T11 {"y Stepper Position"=0, "z Stepper Position"=0} -> [w205]
    shift-right: [w200] -> _
    shift-left: T10 {"Yaw"=0.0, "Compass"=0.0} -> [w202]
    shift-right: [w197] -> _
    shift-left: T9 {"Time up flag"=FALSE, "SET TIME TO CHECK"=0.0} -> [w199]
    shift-right: [w195] -> _
    shift-left: T8 {"yStepper desired"=0} -> [w196]
    stop <- w224 stop-if-true
    # ">>> yStepper command>>>"
    # ">>True Stop Next State >>"
    # "Stays in Task 5_A until stepper reaches desired \nheight"
    # ">>Error  >>"
    # ">>Timeout>>"
    # ">>Action states Queue Reference >>"
    # ">>State Logic Queue Reference >>"
    # "TOP LEVEL BASELINE (MAIN PROCESSING LOOP)"
    n57 = Dequeue Element(queue=w237, timeout in ms (-1)=0, error in (no error)=w235) -> (queue out=w229:refnum<queue>, element=w236:string, error out=w230:errorcluster)  [unwired: 1 out]
    "Action State" <- w236
    n58 = Wait (ms)(milliseconds to wait=u32 50) -> ()  [unwired: 1 out]
    n59 = case shown="\"CAM ACQ\"" w236 {
      tunnel: [_ _ _ _ _ _ _ _ _ _ _ _ _ _ _ _ 0 w1102 _ _ _ _ _ _ _ _ _ _ _ _ _ _ _ _ _ _ _] -> w232
      tunnel: w229 -> [_ _ _ _ _ _ _ _ _ _ _ _ _ _ _ _ _ _ _ _ _ _ _ _ _ _ _ _ _ _ _ _ _ _ _ _ _]
      tunnel: w228 -> [w918 w926 w937 w948 w958 w968 w979 w990 w1000 w1006 w1020 w1033 w1043 w1051 w1075 w1084 w1094 w1103 w1111 w1119 w1148 w1158 w1165 w1173 w1185 w1197 w1216 w1227 w1233 w1242 w1251 w1260 w1268 w1283 w1288 w1299 w1309]
      tunnel: [w918 w926 w937 w948 w958 w968 w979 w990 w1000 w1006 w1020 w1034 w1043 w1051 w1076 w1084 w1094 w1103 w1111 w1119 w1147 w1158 w1165 w1173 w1185 w1197 w1216 w1227 w1233 w1242 w1251 w1260 w1268 w1283 w1288 w1299 w1309] -> w227
      tunnel: [TRUE TRUE _ _ _ _ _ _ _ _ _ _ _ _ _ _ _ _ _ _ _ _ _ _ _ _ _ _ _ _ _ _ _ _ _ _ _] -> w224
      tunnel: w222 -> [w916 w924 w936 w947 w957 w967 w978 w989 w999 w1005 w1019 w1032 w1042 w1050 w1074 w1083 w1091 w1100 w1110 w1118 w1146 w1157 w1164 w1172 w1179 w1191 w1215 w1222 w1232 w1241 w1250 w1259 w1267 w1282 w1287 w1298 w1308]
      tunnel: [_ _ _ _ _ _ _ _ _ _ _ _ _ _ _ _ _ TRUE _ _ _ _ _ _ _ _ _ _ _ _ _ _ _ _ _ _ _] -> w221
      tunnel: [w916 w924 w936 w947 w957 w967 w978 w989 w999 w1005 w1019 w1032 w1042 w1050 w1074 w1083 w1091 w1100 w1110 w1118 w1146 w1157 w1164 w1172 w1179 w1191 w1215 w1222 w1232 w1241 w1250 w1259 w1267 w1282 w1287 w1298 w1308] -> w220
      tunnel: w217 -> [w915 w923 w935 w946 w956 w966 w977 w988 w998 w1007 w1018 w1031 w1044 w1052 w1073 w1085 w1090 w1099 w1112 w1120 w1136 w1156 w1167 w1174 w1186 w1198 w1217 w1228 w1235 w1244 w1253 w1262 w1270 w1285 w1290 w1301 w1311]
      tunnel: [w915 w923 w935 w946 w956 w966 w977 w988 w998 w1007 w1017 w1031 w1044 w1052 w1072 w1085 w1090 w1099 w1112 w1120 w1135 w1156 w1167 w1174 w1186 w1198 w1217 w1228 w1235 w1244 w1253 w1262 w1270 w1285 w1290 w1301 w1311] -> w216
      tunnel: w210 -> [w910 _ _ _ _ _ _ _ _ _ _ _ _ _ _ _ _ _ _ _ _ _ _ _ _ _ w1210 _ _ _ _ _ _ _ _ _ _]
      tunnel: w209 -> [_ _ _ _ _ _ _ _ _ _ _ _ _ _ _ _ _ _ _ _ _ _ _ _ _ _ w1209 _ _ _ _ _ _ _ _ _ _]
      tunnel: w208 -> [w914 w922 w934 w945 w955 w965 w976 w987 w996 w1004 w1016 w1030 w1036 w1049 w1064 w1082 w1089 w1098 w1109 w1117 w1141 w1154 w1166 w1171 w1178 w1190 w1208 w1221 w1234 w1243 w1252 w1261 w1269 w1284 w1289 w1300 w1310]
      tunnel: [w914 w922 w934 w945 w955 w965 w976 w987 w996 w1004 w1016 w1030 w1036 w1049 w1063 w1082 w1089 w1098 w1109 w1117 w1140 w1154 w1166 w1171 w1178 w1190 w1202 w1221 w1234 w1243 w1252 w1261 w1269 w1284 w1289 w1300 w1310] -> w207
      tunnel: w205 -> [w913 w921 w933 w944 w954 w964 w975 w986 w995 w1003 w1015 w1029 w1045 w1048 w1069 w1081 w1088 w1097 w1108 w1116 w1131 w1153 w1163 w1170 w1177 w1189 w1201 w1220 w1231 w1240 w1249 w1258 w1271 w1281 w1291 w1302 w1312]
      tunnel: [w913 w921 w933 w944 w954 w964 w975 w986 w995 w1003 w1015 w1029 w1045 w1048 w1068 w1081 w1088 w1097 w1108 w1116 w1130 w1153 w1163 w1170 w1177 w1189 w1201 w1220 w1231 w1240 w1249 w1258 w1271 w1280 w1291 w1302 w1312] -> w204
      tunnel: w202 -> [w912 w920 w928 w939 w949 w963 w970 w981 w994 w1002 w1009 w1022 w1040 w1047 w1059 w1080 w1087 w1096 w1107 w1115 w1127 w1152 w1160 w1169 w1176 w1188 w1200 w1219 w1230 w1237 w1246 w1255 w1272 w1275 w1292 w1303 w1313]
      tunnel: [w912 w920 w928 w939 w949 w963 w970 w981 w994 w1002 w1009 w1022 w1039 w1047 w1058 w1080 w1087 w1096 w1107 w1115 w1126 w1152 w1160 w1169 w1176 w1188 w1200 w1219 w1230 w1237 w1246 w1255 w1272 w1275 w1292 w1303 w1313] -> w201
      tunnel: w199 -> [w909 w919 w929 w940 w950 w959 w971 w982 w991 w1001 w1008 w1021 w1035 w1046 w1053 w1077 w1086 w1095 w1106 w1113 w1124 w1150 w1159 w1168 w1175 w1187 w1199 w1218 w1229 w1236 w1245 w1254 w1273 w1274 w1286 w1296 w1306]
      tunnel: [w909 w919 w929 w940 w950 w959 w971 w982 w991 w1001 w1008 w1021 w1035 w1046 w1053 w1077 w1086 w1095 w1106 w1113 w1123 w1150 w1159 w1168 w1175 w1187 w1199 w1218 w1229 w1236 w1245 w1254 w1273 w1274 w1286 w1294 w1305] -> w198
      tunnel: w196 -> [_ _ _ _ _ _ _ _ _ _ _ _ _ _ _ _ _ _ _ _ _ _ _ _ _ _ _ _ _ _ _ _ w1264 _ _ _ _]
      frame "Exit" {
        # ">>State Logic  >>"
        # ">>> Time cluster >>>"
        # ">>> Yaw >>>"
        # ">>> Stepper position >>>"
        # ">>> Encoders >>>"
        # ">>> Object detection >>>"
        # ">>> Ultrasonic Sensors Detect >>>"
        n60 = call "Imaq Dispose"("All Images? (No)"=TRUE, "Image"=w910) -> ()  [unwired: 4 in, 1 out]
      }
      frame "----Movement States----" {
        # ">>State Logic  >>"
        # ">>> Time cluster >>>"
        # ">>> Yaw >>>"
        # ">>> Stepper position >>>"
        # ">>> Encoders >>>"
        # ">>> Object detection >>>"
        # ">>> Ultrasonic Sensors Detect >>>"
      }
      frame "FORWARD" {
        # ">>> Time cluster >>>"
        # ">>> Yaw >>>"
        # ">>> Stepper position >>>"
        # ">>> Encoders >>>"
        # ">>> Object detection >>>"
        # ">>> Ultrasonic Sensors Detect >>>"
        n61 = Unbundle By Name(w928) -> ("Yaw"=w927:dbl)
        n62 = call "Motor Control NO PID AE Ver.vi"("Direction"=MOTOR_CONTROL_NO_PID_AE_DIRECTIONS_type_def."y-axis movement", "AE Mode"=MOTOR_CONTROL_NO_PID_AE_DATA_ENTRY_MODE_Type_def."Write to motors", "Speed"=0.5, "Yaw"=w927) -> ()  [unwired: 1 in, 2 out]
      }
      frame "LEFT" {
        # ">>State Logic  >>"
        # ">>> Time cluster >>>"
        # ">>> Yaw >>>"
        # ">>> Stepper position >>>"
        # ">>> Encoders >>>"
        # ">>> Object detection >>>"
        # ">>> Ultrasonic Sensors Detect >>>"
        n63 = Unbundle By Name(w939) -> ("Yaw"=w938:dbl)
        n64 = call "Motor Control NO PID AE Ver.vi"("Direction"=MOTOR_CONTROL_NO_PID_AE_DIRECTIONS_type_def."x-axis movement", "AE Mode"=MOTOR_CONTROL_NO_PID_AE_DATA_ENTRY_MODE_Type_def."Write to motors", "Speed"=-0.5, "Yaw"=w938) -> ()  [unwired: 1 in, 2 out]
      }
      frame "R-ACW" {
        n65 = call "Motor Control NO PID AE Ver.vi"("Direction"=MOTOR_CONTROL_NO_PID_AE_DIRECTIONS_type_def."Rotate", "AE Mode"=MOTOR_CONTROL_NO_PID_AE_DATA_ENTRY_MODE_Type_def."Write to motors", "Speed"=0.5) -> ()  [unwired: 2 in, 2 out]
      }
      frame "R-CW" {
        (unwired) -0.2 ("Speed")
        n66 = call "Motor Control NO PID AE Ver.vi"("Direction"=MOTOR_CONTROL_NO_PID_AE_DIRECTIONS_type_def."Rotate", "AE Mode"=MOTOR_CONTROL_NO_PID_AE_DATA_ENTRY_MODE_Type_def."Write to motors", "Speed"=-0.5) -> ()  [unwired: 2 in, 2 out]
      }
      frame "RIGHT" {
        n67 = Unbundle By Name(w970) -> ("Yaw"=w969:dbl)
        n68 = call "Motor Control NO PID AE Ver.vi"("Direction"=MOTOR_CONTROL_NO_PID_AE_DIRECTIONS_type_def."x-axis movement", "AE Mode"=MOTOR_CONTROL_NO_PID_AE_DATA_ENTRY_MODE_Type_def."Write to motors", "Speed"=-0.5, "Yaw"=w969) -> ()  [unwired: 1 in, 2 out]
      }
      frame "REVERSE" {
        n69 = Unbundle By Name(w981) -> ("Yaw"=w980:dbl)
        n70 = call "Motor Control NO PID AE Ver.vi"("Direction"=MOTOR_CONTROL_NO_PID_AE_DIRECTIONS_type_def."y-axis movement", "AE Mode"=MOTOR_CONTROL_NO_PID_AE_DATA_ENTRY_MODE_Type_def."Write to motors", "Speed"=-0.5, "Yaw"=w980) -> ()  [unwired: 1 in, 2 out]
      }
      frame "STOP" {
        n71 = Wait (ms)(milliseconds to wait=u32 500) -> ()  [unwired: 1 out]
        n72 = call "Motor Control NO PID AE Ver.vi"("Direction"=MOTOR_CONTROL_NO_PID_AE_DIRECTIONS_type_def."Stop", "AE Mode"=MOTOR_CONTROL_NO_PID_AE_DATA_ENTRY_MODE_Type_def."Write to motors") -> ()  [unwired: 3 in, 2 out]
      }
      frame "----SENSOR READING---- " {
      }
      frame "READ ENCODERS" {
        # ">>> Time cluster >>>"
        # ">>> Yaw >>>"
        # ">>> Stepper position >>>"
        # ">>> Object detection >>>"
        # ">>> Current encoder distance >>>"
        # ">>> Ultrasonic Sensors Detect >>>"
        n73 = call "Motor Control NO PID AE Ver.vi"("AE Mode"=MOTOR_CONTROL_NO_PID_AE_DATA_ENTRY_MODE_Type_def."Read from Encoders") -> ("Speed & distance"=w1013:T1)  [unwired: 4 in, 1 out]
        n74 = Unbundle By Name(w1013) -> ("xDistance"=w1012:dbl, "yDistance"=w1011:dbl, "wDistance"=w1010:dbl)
        n75 = Bundle By Name(cluster=w1018, "xDistance"=w1012, "yDistance"=w1011, "wDistance"=w1010) -> (w1017:T15)
      }
      frame "READ ULTRASONIC" {
        (unwired) navX_type_def."Read Values" ("Mode")
        (unwired) MOTOR_CONTROL_NO_PID_Type_Def."Latch" ("Direction")
        # ">>> Ultrasonic Sensors Detect >>>"
        # ">>> Object detection >>>"
        # ">>> Encoders >>>"
        # ">>> Stepper position >>>"
        # ">>> Yaw >>>"
        n76 = call "Arduino Interfacing VI.vi"("AE Mode"=Arduino_Interfacing."Read From Arduino") -> ("Arduino Data"=w1027:T4)  [unwired: 3 in, 1 out]
        n77 = Unbundle By Name(w1027) -> ("PING A"=w1026:u8, "PING B"=w1025:u8, "PING C"=w1024:u8, "PING D"=w1023:u8)
        n78 = Bundle By Name(cluster=w1033, "PING_A"=w1026, "PING_B"=w1025, "PING_C"=w1024, "PING_D"=w1023) -> (w1034:T14)
      }
      frame "READ YAW" {
        # ">>> Yaw >>>"
        # ">>> Ultrasonic Sensors Detect >>>"
        # ">>> Object detection >>>"
        # ">>> Encoders >>>"
        # ">>> Stepper position >>>"
        n79 = call "navX reading VI.vi"("Mode"=navX_type_def."Read Values") -> ("NavX Readings"=w1038:T3)  [unwired: 2 in, 3 out]
        n80 = Unbundle By Name(w1038) -> ("Yaw"=w1037:dbl)
        n81 = Bundle By Name(cluster=w1040, "Yaw"=w1037) -> (w1039:T10)
      }
      frame "----SYSTEM MODES----" {
        (unwired) I2C_MASTER_Type_Def."Last State" ("Arduino Mode")
        # ">>> Object detection >>>"
        # ">>> Yaw >>>"
        # ">>> Ultrasonic Sensors Detect >>>"
        # ">>> Encoders >>>"
        # ">>> Stepper position >>>"
      }
      frame "INIT" {
        w1070 = u8 0
        w1071 = 0.0
        # ">>> Time cluster >>>"
        # ">>> Object detection >>>"
        # ">>> Yaw >>>"
        # ">>> Ultrasonic Sensors Detect >>>"
        # ">>> Encoders >>>"
        # ">>> Stepper position >>>"
        # ">>State Logic  >>"
        n82 = call "Arduino Interfacing VI.vi"("AE Mode"=Arduino_Interfacing."Initialize") -> ()  [unwired: 3 in, 2 out]
        n83 = call "FGV Bool.vi"("Init/Read/Write State"=States_for_Action_Engine."Initialize") -> ()  [unwired: 2 in, 2 out]
        n84 = call "Motor Control NO PID AE Ver.vi"("AE Mode"=MOTOR_CONTROL_NO_PID_AE_DATA_ENTRY_MODE_Type_def."Initialize") -> ()  [unwired: 4 in, 2 out]
        n85 = call "Elasped Timer.vi"("Action"=Control."Initialize") -> ()  [unwired: 7 in, 4 out]
        n86 = Bundle By Name(cluster=w1064, "Recognized Object"=FALSE, "Object X coordinate"=0.0, "Object Y coordinate"=0.0) -> (w1063:T13)
        n87 = Bundle By Name(cluster=w1069, "y Stepper Position"=u8 0, "z Stepper Position"=u8 0) -> (w1068:T11)
        n88 = Bundle By Name(cluster=w1073, "xDistance"=w1071, "yDistance"=w1071, "wDistance"=w1071) -> (w1072:T15)
        n89 = Bundle By Name(cluster=w1075, "PING_A"=w1070, "PING_B"=w1070, "PING_C"=w1070, "PING_D"=w1070) -> (w1076:T14)
        n90 = Bundle By Name(cluster=w1059, "Yaw"=0.0) -> (w1058:T10)
      }
      frame "ARDUINO - ULTRASONIC" {
        # ">>> Object detection >>>"
        # ">>> Yaw >>>"
        # ">>> Ultrasonic Sensors Detect >>>"
        # ">>> Encoders >>>"
        # ">>> Stepper position >>>"
        # ">>State Logic  >>"
        n91 = call "Arduino Interfacing VI.vi"("Data to Write"=I2C_MASTER_WRITE_NEW_Type_Def."Ultrasonic sensors", "AE Mode"=Arduino_Interfacing."Write to Arduino") -> ()  [unwired: 2 in, 2 out]
      }
      frame "NAVX CALIBRATE" {
        # ">>> Object detection >>>"
        # ">>> Yaw >>>"
        # ">>> Ultrasonic Sensors Detect >>>"
        # ">>> Encoders >>>"
        # ">>> Stepper position >>>"
        # ">>State Logic  >>"
        # "Adds a 15 second delay to the startup process \nfor the NavX to calibrate"
        n92 = Wait (ms)(milliseconds to wait=u32 5000) -> ()  [unwired: 1 out]
      }
      frame "NO ACTION", Default {
        (unwired) u8 0 ("y Stepper value")
        (unwired) TRUE ("Latch")
        (unwired) navX_type_def."Read Values" ("Mode")
        (unwired) MOTOR_CONTROL_NO_PID_Type_Def."Latch" ("Direction")
        # ">>> Object detection >>>"
        # ">>> Yaw >>>"
        # ">>> Ultrasonic Sensors Detect >>>"
        # ">>> Encoders >>>"
        # ">>> Stepper position >>>"
        # ">>State Logic  >>"
        n93 = case shown="4" w1100 {
          tunnel: [0 100] -> w1102
          frame 1, Default {
          }
          frame 4 {
          }
        }
      }
      frame "----RESET CASES----" {
        (unwired) I2C_MASTER_Type_Def."Last State" ("Arduino Mode")
        # ">>> Object detection >>>"
        # ">>> Yaw >>>"
        # ">>> Ultrasonic Sensors Detect >>>"
        # ">>> Encoders >>>"
        # ">>> Stepper position >>>"
        # ">>State Logic  >>"
      }
      frame "RESET ENCODERS" {
        # ">>> Object detection >>>"
        # ">>> Yaw >>>"
        # ">>> Ultrasonic Sensors Detect >>>"
        # ">>> Encoders >>>"
        # ">>> Stepper position >>>"
        # ">>State Logic  >>"
        n94 = call "Motor Control NO PID AE Ver.vi"("AE Mode"=MOTOR_CONTROL_NO_PID_AE_DATA_ENTRY_MODE_Type_def."Reset Encoders") -> ()  [unwired: 4 in, 2 out]
      }
      frame "RESET FLAGS" {
        (unwired) I2C_MASTER_Type_Def."Last State" ("Arduino Mode")
        # "Resets any software variables\nand/or non-critical states"
        n95 = Wait (ms)(milliseconds to wait=u32 20) -> ()  [unwired: 1 out]
        n96 = Bundle By Name(cluster=w1124, "Time up flag"=FALSE, "SET TIME TO CHECK"=0.0) -> (w1123:T9)
        n97 = Bundle By Name(cluster=w1141, "Recognized Object"=FALSE, "Object X coordinate"=0.0, "Object Y coordinate"=0.0) -> (w1140:T13)
        n98 = Bundle By Name(cluster=w1131, "y Stepper Position"=u8 0, "z Stepper Position"=u8 0) -> (w1130:T11)
        n99 = Bundle By Name(cluster=w1136, "xDistance"=0.0, "yDistance"=0.0, "wDistance"=0.0) -> (w1135:T15)
        n100 = Bundle By Name(cluster=w1148, "PING_A"=u8 0, "PING_B"=u8 0, "PING_C"=u8 0, "PING_D"=u8 0) -> (w1147:T14)
        n101 = Bundle By Name(cluster=w1127, "Yaw"=0.0) -> (w1126:T10)
      }
      frame "RESET YAW" {
        n102 = Wait (ms)(milliseconds to wait=u32 100) -> ()  [unwired: 1 out]
        n103 = call "navX reading VI.vi"("Mode"=navX_type_def."Zero Yaw") -> ()  [unwired: 2 in, 4 out]
      }
      frame "RESET ARM" {
        n104 = call "Arduino Interfacing VI.vi"("Data to Write"=I2C_MASTER_WRITE_NEW_Type_Def."Soft Reset", "AE Mode"=Arduino_Interfacing."Write to Arduino") -> ()  [unwired: 2 in, 2 out]
      }
      frame "--------CAM STATES-------" {
      }
      frame "OPEN LOG CAM" {
        n105 = call "Low-Level Grab.vi"("States"=State_control."Initialise", "Session In"=T30 "cam0") -> ("error out"=w1181:errorcluster, "Session Out"=w1182:T30)  [unwired: 7 in, 1 out]
        n106 = call "Low-Level Grab.vi"("error in (no error)"=w1181, "States"=State_control."Start camera", "Session In"=w1182) -> ()  [unwired: 6 in, 3 out]
      }
      frame "OPEN LIFE CAM" {
        (unwired) MOTOR_CONTROL_NO_PID_Type_Def."Latch" ("Direction")
        (unwired) navX_type_def."Read Values" ("Mode")
        n107 = call "Low-Level Grab.vi"("States"=State_control."Initialise", "Session In"=T30 "cam1") -> ("error out"=w1193:errorcluster, "Session Out"=w1194:T30)  [unwired: 7 in, 1 out]
        n108 = call "Low-Level Grab.vi"("error in (no error)"=w1193, "States"=State_control."Start camera", "Session In"=w1194) -> ()  [unwired: 6 in, 3 out]
      }
      frame "CAM ACQ" {
        # ">>> Yaw >>>"
        # ">>> Stepper position >>>"
        # ">>> Encoders >>>"
        # ">>> Object detection >>>"
        # ">>> Ultrasonic Sensors Detect >>>"
        # "Object detection"
        n109 = call "Low-Level Grab.vi"("error in (no error)"=w1209, "States"=State_control."Continuous Acquisition ") -> ("error out"=w1212:errorcluster, "Image Out"=w1213:T23)  [unwired: 7 in, 1 out]
        n110 = call "Object Detection SubVI.vi"("Error In"=w1212, "Mode"="Object recognition mode", "Image Dest"=w1210, "Image in"=w1213) -> ("Object Center Coordinates"=w1207:cluster{"x":sgl, "y":sgl}, "Object detection cluster"=w1204:T2)  [unwired: 2 out]
        "Object detection cluster" <- w1204
        "Object Center Coordinates" <- w1207
        n111 = Unbundle By Name(w1204) -> ("Object detected?"=w1203:bool)
        n112 = Unbundle By Name(w1207) -> ("x"=w1206:sgl, "y"=w1205:sgl)
        n113 = Bundle By Name(cluster=w1208, "Recognized Object"=w1203, "Object X coordinate"=w1206, "Object Y coordinate"=w1205) -> (w1202:T13)
      }
      frame "CAM CLOSE" {
        n114 = call "Low-Level Grab.vi"("States"=State_control."Stop camera") -> ("error out"=w1224:errorcluster, "Session Out"=w1225:T30)  [unwired: 8 in, 1 out]
        n115 = call "Low-Level Grab.vi"("error in (no error)"=w1224, "States"=State_control."Dispose all", "Session In"=w1225) -> ()  [unwired: 6 in, 3 out]
      }
      frame "-----ARM ACTIONS-----" {
      }
      frame "CLOSE CLAW" {
        n116 = call "Arduino Interfacing VI.vi"("Data to Write"=I2C_MASTER_WRITE_NEW_Type_Def."Close Claw", "AE Mode"=Arduino_Interfacing."Write to Arduino") -> ()  [unwired: 2 in, 2 out]
      }
      frame "OPEN CLAW" {
        n117 = call "Arduino Interfacing VI.vi"("Data to Write"=I2C_MASTER_WRITE_NEW_Type_Def."Open Claw", "AE Mode"=Arduino_Interfacing."Write to Arduino") -> ()  [unwired: 2 in, 2 out]
      }
      frame "Z STEPPER CAM HEIGHT" {
        n118 = call "Arduino Interfacing VI.vi"("Data to Write"=I2C_MASTER_WRITE_NEW_Type_Def."zStepper 8k", "AE Mode"=Arduino_Interfacing."Write to Arduino") -> ()  [unwired: 2 in, 2 out]
      }
      frame "Y STEPPER CONTROL" {
        # ">>> yStepper command>>>"
        # ">>> Time cluster >>>"
        # ">>> Yaw >>>"
        # ">>> Stepper position >>>"
        # ">>> Encoders >>>"
        # ">>> Object detection >>>"
        # ">>> Ultrasonic Sensors Detect >>>"
        n119 = Unbundle By Name(w1264) -> ("yStepper desired"=w1263:u8)
        n120 = call "Arduino Interfacing VI.vi"("y Stepper value"=w1263, "Data to Write"=I2C_MASTER_WRITE_NEW_Type_Def."yStepper control", "AE Mode"=Arduino_Interfacing."Write to Arduino") -> ()  [unwired: 1 in, 2 out]
      }
      frame "READ STEPPER VALUES" {
        # ">>State Logic  >>"
        # ">>> Time cluster >>>"
        # ">>> Yaw >>>"
        # ">>> Stepper position >>>"
        # ">>> Encoders >>>"
        # ">>> Object detection >>>"
        # ">>> Ultrasonic Sensors Detect >>>"
        n121 = call "Arduino Interfacing VI.vi"("AE Mode"=Arduino_Interfacing."Read From Arduino") -> ("Arduino Data"=w1278:T4)  [unwired: 3 in, 1 out]
        n122 = Unbundle By Name(w1278) -> ("y Stepper Position"=w1277:u8, "z Stepper Position"=w1276:u8)
        n123 = Bundle By Name(cluster=w1281, "y Stepper Position"=w1277, "z Stepper Position"=w1276) -> (w1280:T11)
      }
      frame " -----TIMING-----" {
        # ">>State Logic  >>"
        # ">>> Time cluster >>>"
        # ">>> Yaw >>>"
        # ">>> Stepper position >>>"
        # ">>> Encoders >>>"
        # ">>> Object detection >>>"
        # ">>> Ultrasonic Sensors Detect >>>"
      }
      frame "SET TIMER" {
        # ">>State Logic  >>"
        # ">>> Time cluster >>>"
        # ">>> Yaw >>>"
        # ">>> Stepper position >>>"
        # ">>> Encoders >>>"
        # ">>> Object detection >>>"
        # ">>> Ultrasonic Sensors Detect >>>"
        n124 = call "Elasped Timer.vi"("Time Setting"=5.0, "Action"=Control."Initialize") -> ()  [unwired: 6 in, 4 out]
        n125 = Bundle By Name(cluster=w1296, "Time up flag"=FALSE) -> (w1294:T9)
      }
      frame "START TIMER" {
        # ">>State Logic  >>"
        # ">>> Time cluster >>>"
        # ">>> Yaw >>>"
        # ">>> Stepper position >>>"
        # ">>> Encoders >>>"
        # ">>> Object detection >>>"
        # ">>> Ultrasonic Sensors Detect >>>"
        n126 = call "Elasped Timer.vi"("Action"=Control."Start") -> ("Time Out?!"=w1304:bool)  [unwired: 7 in, 3 out]
        n127 = Bundle By Name(cluster=w1306, "Time up flag"=w1304) -> (w1305:T9)
      }
    }
    "State Logic" <- w220
    n128 = local read "TASK ENABLE"() -> (w214:bool)
    n129 = Not(x=w214) -> (.not. x?=w213:bool)
    n130 = case shown="True" w221 {
      tunnel: w225 -> [w248 w277]
      tunnel: w229 -> [w244 w279]
      tunnel: [w248 w277] -> w234
      tunnel: [w244 w280] -> w233
      tunnel: w230 -> [_ w275]
      tunnel: w232 -> [_ w276]
      tunnel: w227 -> [w247 w282]
      tunnel: [w247 w282] -> w226
      tunnel: "STOP TASK" -> [_ w265]
      tunnel: w220 -> [w246 w281]
      tunnel: [w246 w278] -> w219
      tunnel: w216 -> [w245 w271]
      tunnel: [w245 w271] -> w215
      tunnel: w213 -> [_ w266]
      tunnel: [w243 w263] -> w212
      tunnel: w211 -> [w243 w262]
      tunnel: w207 -> [w242 w259]
      tunnel: [w242 w259] -> w206
      tunnel: w204 -> [w241 w255]
      tunnel: [w241 w255] -> w203
      tunnel: w201 -> [w240 w253]
      tunnel: [w240 w253] -> w200
      tunnel: w198 -> [w239 w251]
      tunnel: [w239 w251] -> w197
      tunnel: w196 -> [w238 w250]
      tunnel: [w238 w249] -> w195
      frame False {
        # ">>> yStepper command>>>"
        # ">>> Time cluster >>>"
        # ">>> Yaw >>>"
        # ">>> Stepper position >>>"
        # ">>> Encoders >>>"
        # ">>> Object detection >>>"
        # ">>> Ultrasonic Sensors Detect >>>"
        # ">>> Time cluster >>>"
        # ">>> Yaw >>>"
        # ">>> Stepper position >>>"
        # ">>> Encoders >>>"
        # ">>> Object detection >>>"
        # ">>> Ultrasonic Sensors Detect >>>"
      }
      frame True {
        # ">>State Logic Queue Reference >>"
        # ">>Timeout>>"
        # ">>> yStepper command>>>"
        # ">>> Time cluster >>>"
        # ">>> Object detection >>>"
        # ">>> Yaw >>>"
        # ">>> Ultrasonic Sensors Detect >>>"
        # ">>> Encoders >>>"
        # ">>> Stepper position >>>"
        # ">>State Logic  >>"
        # ">>True Stop Next State >>"
        # ">>Action Queue>>"
        # ">> Manual override >>"
        # ">>> Time cluster >>>"
        # ">>> Yaw >>>"
        # ">>> Stepper position >>>"
        # ">>> Encoders >>>"
        # ">>> Object detection >>>"
        # ">>> Ultrasonic Sensors Detect >>>"
        # ">>Action Queue>>"
        # ">>State Logic Queue Reference >>"
        n131 = Or(x=w265, y=w266) -> (x .or. y?=w264:bool)
        n132 = Unbundle By Name(w251) -> ("Time up flag"=w252:bool)
        "Time up flag" <- w252
        n133 = Unbundle By Name(w253) -> ("Yaw"=w254:dbl)
        n134 = Unbundle By Name(w255) -> ("y Stepper Position"=w257:u8, "z Stepper Position"=w256:u8)
        n135 = Unbundle By Name(w271) -> ("xDistance"=w268:dbl, "yDistance"=w269:dbl, "wDistance"=w270:dbl)
        n136 = Unbundle By Name(w259) -> ("Recognized Object"=w258:bool, "Object X coordinate"=w261:dbl, "Object Y coordinate"=w260:dbl)
        n137 = Unbundle By Name(w282) -> ("PING_A"=w274:u8, "PING_B"=w273:u8, "PING_C"=w272:u8, "PING_D"=w267:u8)
        n138 = case shown="15" w281 {
          tunnel: [w285 w289 w301 w309 w369 w382 w419 w466 w511 w569 w607 w662 w703 w745 w795 w838 w880] -> w280
          tunnel: w279 -> [w285 w292 w302 w312 w371 w383 w420 w467 w517 w562 w611 w652 w706 w751 w794 w833 w871]
          tunnel: [State_Type_Definitions."Idle" ("Enum") State_Type_Definitions."Idle" ("Enum") w297 w311 State_Type_Definitions."Shutdown" ("Enum") w384 w422 w465 w512 w568 w608 w661 w704 w752 w796 w839 w872] -> w278
          tunnel: w277 -> [_ _ w300 w315 _ w389 w432 w474 w516 w566 w612 w659 w698 w750 w792 w836 w879]
          tunnel: w276 -> [_ _ _ w314 _ w388 w431 w473 w515 w565 w604 w658 w697 w749 w791 w835 w877]
          tunnel: w275 -> [_ _ w299 w310 _ w387 w430 w472 w514 w564 w603 w660 w699 w748 w790 w834 w878]
          tunnel: w264 -> [_ _ _ _ _ w381 w421 w469 w510 w567 w609 w653 w707 w746 w793 w837 w875]
          tunnel: w274 -> [_ _ _ _ _ _ _ _ _ _ _ _ _ _ _ _ _]
          tunnel: w273 -> [_ _ _ _ _ _ w428 _ w508 w557 w614 _ _ _ _ _ _]
          tunnel: w272 -> [_ _ _ _ _ _ w427 _ w509 w558 w613 _ _ _ _ _ _]
          tunnel: w270 -> [_ _ _ _ _ _ _ w471 _ _ _ _ _ _ _ _ _]
          tunnel: w269 -> [_ _ _ _ _ w380 _ _ _ _ _ _ _ _ _ _ _]
          tunnel: w268 -> [_ _ _ _ _ _ _ _ _ w553 _ _ _ _ _ _ _]
          tunnel: w267 -> [_ _ _ _ _ _ _ _ _ _ _ _ _ _ _ _ _]
          tunnel: [State_Type_Definitions."Idle" ("Enum") State_Type_Definitions."Idle" ("Enum") State_Type_Definitions."Idle" ("Enum") State_Type_Definitions."Idle" ("Enum") State_Type_Definitions."Shutdown" ("Enum") w377 w418 w462 w503 w552 w606 w663 w705 w744 w797 w840 w873] -> w263
          tunnel: w262 -> [_ _ w297 _ _ _ _ _ _ _ _ _ _ _ _ _ _]
          tunnel: w258 -> [_ _ _ _ _ _ _ _ _ _ _ _ w702 _ _ _ w874]
          tunnel: w261 -> [_ _ _ _ _ _ _ _ _ _ _ _ _ _ _ _ _]
          tunnel: w260 -> [_ _ _ _ _ _ _ _ _ _ _ _ _ w743 w782 _ _]
          tunnel: w257 -> [_ _ _ _ _ _ _ _ _ _ _ _ _ _ w785 _ _]
          tunnel: w256 -> [_ _ _ _ _ _ _ _ _ _ _ w656 _ _ _ w832 _]
          tunnel: w254 -> [_ _ _ _ _ _ _ _ _ _ _ _ _ _ _ _ _]
          tunnel: w252 -> [_ _ _ _ _ _ _ _ _ _ _ _ w701 _ _ _ _]
          tunnel: w250 -> [w283 w287 w296 w307 w367 w376 w417 w461 w502 w550 w602 w651 w695 w739 w788 w829 w870]
          tunnel: [w283 w287 w296 w307 w367 w376 w417 w461 w502 w550 w602 w651 w695 w739 w787 w829 w870] -> w249
          frame 0 {
            # ">>> yStepper command>>>"
          }
          frame 1 {
            # ">>> yStepper command>>>"
            n139 = for {
              shift-right: [w295] -> w289
              shift-left: w292 -> [w294]
              tunnel: string[] ["INIT", "RESET ARM", "RESET FLAGS", "RESET YAW", "NAVX CALIBRATE"] -> [w293] mode=indexing
              n140 = Enqueue Element(queue=w294, element=w293) -> (queue out=w295:refnum<queue>)  [unwired: 2 in, 2 out]
            }
          }
          frame 3 {
            # ">>> yStepper command>>>"
            n141 = Flush Queue(queue=w300, error in (no error)=w299) -> ()  [unwired: 3 out]
            n142 = for {
              shift-right: [w306] -> w301
              shift-left: w302 -> [w305]
              tunnel: string[] ["STOP", "RESET ENCODERS", "RESET YAW", "RESET ARM", "RESET FLAGS", "CAM CLOSE"] -> [w304] mode=indexing
              n143 = Enqueue Element(queue=w305, element=w304) -> (queue out=w306:refnum<queue>)  [unwired: 2 in, 2 out]
            }
          }
          frame 4, Default {
            (unwired) TRUE ("Green LED")
            # ">>> yStepper command>>>"
            n144 = Dequeue Element(queue=w315, timeout in ms (-1)=w314, error in (no error)=w310) -> (element=w313:T7)  [unwired: 3 out]
            n145 = case shown="\"Start Task 5\"" w313 {
              tunnel: [w317 w324 w331 w338 w345 w352 w359 w361] -> w309
              tunnel: w312 -> [w318 w325 w332 w339 w346 w353 w359 w362]
              tunnel: [State_Type_Definitions."Task 1" ("Enum") State_Type_Definitions."Task 2" ("Enum") State_Type_Definitions."Task 3" ("Enum") State_Type_Definitions."Task 4_A" ("Enum") State_Type_Definitions."Task 5_A" ("Enum") State_Type_Definitions."Task 6_A" ("Enum") State_Type_Definitions."Idle" ("Enum") State_Type_Definitions."Shutdown" ("Enum")] -> w311
              frame "Start Task 1" {
                n146 = for {
                  shift-right: [w322] -> w317
                  shift-left: w318 -> [w321]
                  tunnel: string[] ["RESET ENCODERS", "RESET YAW", "FORWARD", "READ ENCODERS"] -> [w320] mode=indexing
                  n147 = Enqueue Element(queue=w321, element=w320) -> (queue out=w322:refnum<queue>)  [unwired: 2 in, 2 out]
                }
              }
              frame "Start Task 2" {
                n148 = for {
                  shift-right: [w329] -> w324
                  shift-left: w325 -> [w328]
                  tunnel: string[] ["RESET ENCODERS", "RESET YAW", "READ ULTRASONIC", "ARDUINO - ULTRASONIC"] -> [w327] mode=indexing
                  n149 = Enqueue Element(queue=w328, element=w327) -> (queue out=w329:refnum<queue>)  [unwired: 2 in, 2 out]
                }
              }
              frame "Start Task 3" {
                n150 = for {
                  shift-right: [w336] -> w331
                  shift-left: w332 -> [w335]
                  tunnel: string[] ["RESET ENCODERS", "READ ENCODERS", "R-ACW"] -> [w334] mode=indexing
                  n151 = Enqueue Element(queue=w335, element=w334) -> (queue out=w336:refnum<queue>)  [unwired: 2 in, 2 out]
                }
              }
              frame "Start Task 4" {
                n152 = for {
                  shift-right: [w343] -> w338
                  shift-left: w339 -> [w342]
                  tunnel: string[] ["STOP", "RESET YAW", "RESET ENCODERS", "READ ULTRASONIC", "ARDUINO - ULTRASONIC", ""] -> [w341] mode=indexing
                  n153 = Enqueue Element(queue=w342, element=w341) -> (queue out=w343:refnum<queue>)  [unwired: 2 in, 2 out]
                }
              }
              frame "Start Task 5" {
                n154 = for {
                  shift-right: [w350] -> w345
                  shift-left: w346 -> [w349]
                  tunnel: string[] ["RESET YAW", "RESET ENCODERS", "READ STEPPER VALUES", "Z STEPPER CAM HEIGHT", "", ""] -> [w348] mode=indexing
                  n155 = Enqueue Element(queue=w349, element=w348) -> (queue out=w350:refnum<queue>)  [unwired: 2 in, 2 out]
                }
              }
              frame "Start Task 6" {
                n156 = for {
                  shift-right: [w357] -> w352
                  shift-left: w353 -> [w356]
                  tunnel: string[] ["Z STEPPER CAM HEIGHT ", "READ STEPPER VALUES", "OPEN LOG CAM", "", "", ""] -> [w355] mode=indexing
                  n157 = Enqueue Element(queue=w356, element=w355) -> (queue out=w357:refnum<queue>)  [unwired: 2 in, 2 out]
                }
              }
              frame "None", Default {
              }
              frame "Exit" {
                n158 = for {
                  shift-right: [w366] -> w361
                  shift-left: w362 -> [w365]
                  tunnel: string[] ["STOP", "RESET ENCODERS", "RESET YAW", "EXIT"] -> [w364] mode=indexing
                  n159 = Enqueue Element(queue=w365, element=w364) -> (queue out=w366:refnum<queue>)  [unwired: 2 in, 2 out]
                }
              }
            }
          }
          frame 5 {
            # ">>> yStepper command>>>"
            n160 = for {
              shift-right: [w375] -> w369
              shift-left: w371 -> [w374]
              tunnel: string[] ["INIT", "RESET ENCODERS", "RESET FLAGS", "EXIT"] -> [w373] mode=indexing
              n161 = Enqueue Element(queue=w374, element=w373) -> (queue out=w375:refnum<queue>)  [unwired: 2 in, 2 out]
            }
          }
          frame 6 {
            # ">>> yStepper command>>>"
            # "Use 250"
            n162 = Dequeue Element(queue=w389, timeout in ms (-1)=w388, error in (no error)=w387) -> (element=w386:T7)  [unwired: 3 out]
            n163 = Greater?(x=w380, y=10000.0) -> (0:w378:bool)
            n164 = Or(x=w378, y=w381) -> (x .or. y?=w385:bool)
            n165 = case shown="\"None\", Default" w386 {
              tunnel: w385 -> [w392 _]
              tunnel: [w396 State_Type_Definitions."True Stop" ("Enum")] -> w384
              tunnel: w383 -> [w393 w411]
              tunnel: [w391 w410] -> w382
              tunnel: [State_Type_Definitions."Idle" ("Enum") State_Type_Definitions."Shutdown" ("Enum")] -> w377
              frame "None", Default {
                n166 = case shown="True" w392 {
                  tunnel: w393 -> [w399 w405]
                  tunnel: [w398 w403] -> w391
                  frame False {
                    n167 = for {
                      shift-right: [w401] -> w398
                      shift-left: w399 -> [w402]
                      tunnel: string[] ["READ ENCODERS", "READ YAW", "FORWARD"] ("element") -> [w400] mode=indexing
                      n168 = Enqueue Element(queue=w402, element=w400) -> (queue out=w401:refnum<queue>)  [unwired: 2 in, 2 out]
                    }
                  }
                  frame True {
                    n169 = for {
                      shift-right: [w407] -> w403
                      shift-left: w405 -> [w408]
                      tunnel: string[] ["RESET YAW", "RESET ENCODERS", "STOP", ""] -> [w406] mode=indexing
                      n170 = Enqueue Element(queue=w408, element=w406) -> (queue out=w407:refnum<queue>)  [unwired: 2 in, 2 out]
                    }
                  }
                }
                n171 = Select(t=State_Type_Definitions."True Stop" ("Enum"), s=w392, f=State_Type_Definitions."Task 1" ("Enum")) -> (s? t:f=w396:u16)
              }
              frame "Exit" {
                n172 = for {
                  shift-right: [w415] -> w410
                  shift-left: w411 -> [w416]
                  tunnel: string[] ["STOP", "RESET ENCODERS", "RESET YAW", ""] -> [w414] mode=indexing
                  n173 = Enqueue Element(queue=w416, element=w414) -> (queue out=w415:refnum<queue>)  [unwired: 2 in, 2 out]
                }
              }
            }
          }
          frame 7 {
            w426 = u8 10 ("y")
            # ">>> yStepper command>>>"
            # ">>Object detected>>"
            n174 = Dequeue Element(queue=w432, timeout in ms (-1)=w431, error in (no error)=w430) -> (element=w429:T7)  [unwired: 3 out]
            n175 = Less?(x=w428, y=w426) -> (x < y?=w425:bool)
            n176 = Less?(x=w427, y=w426) -> (x < y?=w424:bool)
            n177 = Or(x=w425, y=w424) -> (x .or. y?=w423:bool)
            "Object detected?" <- w423
            n178 = case shown="\"None\", Default" w429 {
              tunnel: w423 -> [w436 _]
              tunnel: [w438 State_Type_Definitions."True Stop" ("Enum")] -> w422
              tunnel: w421 -> [w437 _]
              tunnel: w420 -> [w435 w455]
              tunnel: [w434 w456] -> w419
              tunnel: [State_Type_Definitions."Idle" ("Enum") State_Type_Definitions."Shutdown" ("Enum")] -> w418
              frame "None", Default {
                n179 = case shown="False" w436 {
                  tunnel: w435 -> [w442 w449]
                  tunnel: [w443 w448] -> w434
                  frame False {
                    n180 = for {
                      tunnel: string[] ["READ ULTRASONIC", "STOP"] ("element") -> [w444] mode=indexing
                      shift-right: [w446] -> w443
                      shift-left: w442 -> [w445]
                      n181 = Enqueue Element(queue=w445, element=w444) -> (queue out=w446:refnum<queue>)  [unwired: 2 in, 2 out]
                    }
                  }
                  frame True {
                    n182 = for {
                      shift-right: [w451] -> w448
                      shift-left: w449 -> [w452]
                      tunnel: string[] ["REVERSE", "READ ULTRASONIC"] -> [w450] mode=indexing
                      n183 = Enqueue Element(queue=w452, element=w450) -> (queue out=w451:refnum<queue>)  [unwired: 2 in, 2 out]
                    }
                  }
                }
                n184 = Select(t=State_Type_Definitions."True Stop" ("Enum"), s=w437, f=State_Type_Definitions."Task 2" ("Enum")) -> (s? t:f=w438:u16)
              }
              frame "Exit" {
                n185 = for {
                  shift-right: [w459] -> w456
                  shift-left: w455 -> [w460]
                  tunnel: string[] ["STOP", "RESET ENCODERS", "RESET YAW", "ARDUINO MODE 0"] -> [w458] mode=indexing
                  n186 = Enqueue Element(queue=w460, element=w458) -> (queue out=w459:refnum<queue>)  [unwired: 2 in, 2 out]
                }
              }
            }
          }
          frame 10 {
            # ">>> yStepper command>>>"
            n187 = Dequeue Element(queue=w474, timeout in ms (-1)=w473, error in (no error)=w472) -> (element=w463:T7)  [unwired: 3 out]
            n188 = Greater?(x=w471, y=150.0) -> (0:w468:bool)
            n189 = Or(x=w468, y=w469) -> (x .or. y?=w464:bool)
            n190 = case shown="\"Exit\"" w463 {
              tunnel: w464 -> [w477 _]
              tunnel: [w481 State_Type_Definitions."True Stop" ("Enum")] -> w465
              tunnel: w467 -> [w478 w497]
              tunnel: [w476 w496] -> w466
              tunnel: [State_Type_Definitions."Idle" ("Enum") State_Type_Definitions."Shutdown" ("Enum")] -> w462
              frame "None", Default {
                n191 = case shown="False" w477 {
                  tunnel: w478 -> [w484 w490]
                  tunnel: [w483 w488] -> w476
                  frame False {
                    n192 = for {
                      shift-right: [w486] -> w483
                      shift-left: w484 -> [w487]
                      tunnel: string[] ["READ ENCODERS", "R-ACW"] ("element") -> [w485] mode=indexing
                      n193 = Enqueue Element(queue=w487, element=w485) -> (queue out=w486:refnum<queue>)  [unwired: 2 in, 2 out]
                    }
                  }
                  frame True {
                    n194 = for {
                      shift-right: [w492] -> w488
                      shift-left: w490 -> [w493]
                      tunnel: string[] ["RESET YAW", "RESET ENCODERS", "STOP", "ARDUINO MODE 0"] -> [w491] mode=indexing
                      n195 = Enqueue Element(queue=w493, element=w491) -> (queue out=w492:refnum<queue>)  [unwired: 2 in, 2 out]
                    }
                  }
                }
                n196 = Select(t=State_Type_Definitions."True Stop" ("Enum"), s=w477, f=State_Type_Definitions."Task 3" ("Enum")) -> (s? t:f=w481:T6)
              }
              frame "Exit" {
                n197 = for {
                  shift-right: [w500] -> w496
                  shift-left: w497 -> [w501]
                  tunnel: string[] ["STOP", "RESET ENCODERS", "RESET YAW", ""] -> [w499] mode=indexing
                  n198 = Enqueue Element(queue=w501, element=w499) -> (queue out=w500:refnum<queue>)  [unwired: 2 in, 2 out]
                }
              }
            }
          }
          frame 11 {
            w507 = 20
            # ">>> yStepper command>>>"
            # ">> Outputs true if object detected >>"
            # ">> Manual override >>"
            n199 = Dequeue Element(queue=w516, timeout in ms (-1)=w515, error in (no error)=w514) -> (element=w513:T7)  [unwired: 3 out]
            n200 = Less?(x=w509, y=w507) -> (x < y?=w505:bool)
            n201 = Less?(x=w508, y=w507) -> (x < y?=w506:bool)
            n202 = And(x=w506, y=w505) -> (x .and. y?=w504:bool)
            "Detect?" <- w504
            n203 = case shown="\"None\", Default" w513 {
              tunnel: [w526 State_Type_Definitions."True Stop" ("Enum")] -> w512
              tunnel: [w524 w545] -> w511
              tunnel: w517 -> [w523 _]
              tunnel: w510 -> [w521 _]
              tunnel: w504 -> [w519 _]
              tunnel: [w518 State_Type_Definitions."Shutdown" ("Enum")] -> w503
              frame "None", Default {
                # ">> WIill proceed to part ii if not manual override >>"
                # ">>If ENABLE or Trigger is set to true>>"
                n204 = Or(x=w519, y=w521) -> (x .or. y?=w520:bool)
                n205 = case shown="False" w520 {
                  tunnel: [w533 w538] -> w524
                  tunnel: w523 -> [w531 w537]
                  frame False {
                    n206 = for {
                      shift-right: [w535] -> w533
                      shift-left: w531 -> [w536]
                      tunnel: string[] ["FORWARD", "ULTRASONIC READ", ""] ("element") -> [w534] mode=indexing
                      n207 = Enqueue Element(queue=w536, element=w534) -> (queue out=w535:refnum<queue>)  [unwired: 2 in, 2 out]
                    }
                  }
                  frame True {
                    n208 = for {
                      shift-right: [w541] -> w538
                      shift-left: w537 -> [w542]
                      tunnel: string[] ["STOP", "RESET ENCODERS", "RESET YAW", "ARDUINO MODE 0"] -> [w540] mode=indexing
                      n209 = Enqueue Element(queue=w542, element=w540) -> (queue out=w541:refnum<queue>)  [unwired: 2 in, 2 out]
                    }
                  }
                }
                n210 = case shown="False" w521 {
                  tunnel: [State_Type_Definitions."True Stop" ("Enum") State_Type_Definitions."True Stop" ("Enum")] -> w522
                  tunnel: [State_Type_Definitions."Task 4_B" ("Enum") State_Type_Definitions."Idle" ("Enum")] -> w518
                  frame False {
                  }
                  frame True {
                  }
                }
                n211 = Select(t=w522, s=w520, f=State_Type_Definitions."Task 4_A" ("Enum")) -> (s? t:f=w526:T6)
              }
              frame "Exit" {
                n212 = for {
                  shift-right: [w548] -> w545
                  shift-left: _ -> [w549]
                  tunnel: string[] ["STOP", "RESET ENCODERS", "RESET YAW", ""] -> [w547] mode=indexing
                  n213 = Enqueue Element(queue=w549, element=w547) -> (queue out=w548:refnum<queue>)  [unwired: 2 in, 2 out]
                }
              }
            }
          }
          frame 12 {
            w561 = 20
            # ">>> yStepper command>>>"
            # ">> Outputs true if 150 mm has been moved >>"
            # ">> Outputs true if sensor not obstructed>>"
            # ">> Manual override >>"
            n214 = Dequeue Element(queue=w566, timeout in ms (-1)=w565, error in (no error)=w564) -> (element=w563:T7)  [unwired: 3 out]
            n215 = Greater?(x=w558, y=w561) -> (0:w559:bool)
            n216 = Greater?(x=w557, y=w561) -> (0:w560:bool)
            n217 = Greater Or Equal?(x=w553, y=80.0) -> (x >= y?=w555:bool)
            n218 = And(x=w560, y=w559) -> (x .and. y?=w554:bool)
            n219 = And(x=w555, y=w554) -> (x .and. y?=w551:bool)
            n220 = case shown="\"None\", Default" w563 {
              tunnel: [w578 State_Type_Definitions."True Stop" ("Enum")] -> w568
              tunnel: [w576 w597] -> w569
              tunnel: w562 -> [w575 _]
              tunnel: w567 -> [w573 _]
              tunnel: w551 -> [w571 _]
              tunnel: [w570 State_Type_Definitions."Shutdown" ("Enum")] -> w552
              frame "None", Default {
                # ">> WIill proceed to part ii if not manual override >>"
                # ">>If ENABLE or Trigger is set to true>>"
                n221 = Or(x=w571, y=w573) -> (x .or. y?=w572:bool)
                n222 = case shown="False" w572 {
                  tunnel: [w585 w590] -> w576
                  tunnel: w575 -> [w583 w589]
                  frame False {
                    n223 = for {
                      shift-right: [w587] -> w585
                      shift-left: w583 -> [w588]
                      tunnel: string[] ["RIGHT", "ULTRASONIC READ", "READ ENCODERS"] ("element") -> [w586] mode=indexing
                      n224 = Enqueue Element(queue=w588, element=w586) -> (queue out=w587:refnum<queue>)  [unwired: 2 in, 2 out]
                    }
                  }
                  frame True {
                    n225 = for {
                      shift-right: [w593] -> w590
                      shift-left: w589 -> [w594]
                      tunnel: string[] ["STOP", "RESET ENCODERS", "RESET YAW", "ARDUINO MODE 0"] -> [w592] mode=indexing
                      n226 = Enqueue Element(queue=w594, element=w592) -> (queue out=w593:refnum<queue>)  [unwired: 2 in, 2 out]
                    }
                  }
                }
                n227 = case shown="True" w573 {
                  tunnel: [State_Type_Definitions."True Stop" ("Enum") State_Type_Definitions."True Stop" ("Enum")] -> w574
                  tunnel: [State_Type_Definitions."Task 4_C" ("Enum") State_Type_Definitions."Idle" ("Enum")] -> w570
                  frame False {
                  }
                  frame True {
                  }
                }
                n228 = Select(t=w574, s=w572, f=State_Type_Definitions."Task 4_B" ("Enum")) -> (s? t:f=w578:T6)
              }
              frame "Exit" {
                n229 = for {
                  shift-right: [w600] -> w597
                  shift-left: _ -> [w601]
                  tunnel: string[] ["STOP", "RESET ENCODERS", "RESET YAW", ""] -> [w599] mode=indexing
                  n230 = Enqueue Element(queue=w601, element=w599) -> (queue out=w600:refnum<queue>)  [unwired: 2 in, 2 out]
                }
              }
            }
          }
          frame 13 {
            w617 = u8 20
            # ">>> yStepper command>>>"
            # ">> Outputs true if object detected >>"
            # ">> Manual override >>"
            n231 = Dequeue Element(queue=w612, timeout in ms (-1)=w604, error in (no error)=w603) -> (element=w605:T7)  [unwired: 3 out]
            n232 = Less?(x=w613, y=w617) -> (x < y?=w615:bool)
            n233 = Less?(x=w614, y=w617) -> (x < y?=w616:bool)
            n234 = And(x=w616, y=w615) -> (x .and. y?=w610:bool)
            n235 = case shown="\"None\", Default" w605 {
              tunnel: [w626 State_Type_Definitions."True Stop" ("Enum")] -> w608
              tunnel: [w624 w646] -> w607
              tunnel: w611 -> [w623 w643]
              tunnel: w609 -> [w621 _]
              tunnel: w610 -> [w619 _]
              tunnel: [w618 State_Type_Definitions."Shutdown" ("Enum")] -> w606
              frame "None", Default {
                # ">> WIill proceed to part ii if not manual override >>"
                # ">>If ENABLE or Trigger is set to true>>"
                n236 = Or(x=w619, y=w621) -> (x .or. y?=w620:bool)
                n237 = case shown="False" w620 {
                  tunnel: [w633 w638] -> w624
                  tunnel: w623 -> [w631 w637]
                  frame False {
                    n238 = for {
                      shift-right: [w635] -> w633
                      shift-left: w631 -> [w636]
                      tunnel: string[] ["FORWARD", "ULTRASONIC READ", ""] ("element") -> [w634] mode=indexing
                      n239 = Enqueue Element(queue=w636, element=w634) -> (queue out=w635:refnum<queue>)  [unwired: 2 in, 2 out]
                    }
                  }
                  frame True {
                    n240 = for {
                      shift-right: [w641] -> w638
                      shift-left: w637 -> [w642]
                      tunnel: string[] ["STOP", "RESET ENCODERS", "RESET YAW", "ARDUINO MODE 0"] -> [w640] mode=indexing
                      n241 = Enqueue Element(queue=w642, element=w640) -> (queue out=w641:refnum<queue>)  [unwired: 2 in, 2 out]
                    }
                  }
                }
                n242 = case shown="True" w621 {
                  tunnel: [State_Type_Definitions."True Stop" ("Enum") State_Type_Definitions."True Stop" ("Enum")] -> w622
                  tunnel: [State_Type_Definitions."Idle" ("Enum") State_Type_Definitions."Idle" ("Enum")] -> w618
                  frame False {
                  }
                  frame True {
                  }
                }
                n243 = Select(t=w622, s=w620, f=State_Type_Definitions."Task 4_C" ("Enum")) -> (s? t:f=w626:T6)
              }
              frame "Exit" {
                n244 = for {
                  shift-right: [w649] -> w646
                  shift-left: w643 -> [w650]
                  tunnel: string[] ["STOP", "RESET ENCODERS", "RESET YAW", ""] -> [w648] mode=indexing
                  n245 = Enqueue Element(queue=w650, element=w648) -> (queue out=w649:refnum<queue>)  [unwired: 2 in, 2 out]
                }
              }
            }
          }
          frame 12 {
            # ">>> yStepper command>>>"
            # ">> Manual override >>"
            n246 = Dequeue Element(queue=w659, timeout in ms (-1)=w658, error in (no error)=w660) -> (element=w657:T7)  [unwired: 3 out]
            n247 = Equal?(x=w656, y=u8 80) -> (x = y?=w654:bool)
            n248 = case shown="\"None\", Default" w657 {
              tunnel: [w670 State_Type_Definitions."True Stop" ("Enum")] -> w661
              tunnel: [w673 w690] -> w662
              tunnel: [State_Type_Definitions."Idle" ("Enum") State_Type_Definitions."Shutdown" ("Enum")] -> w663
              tunnel: w654 -> [w669 _]
              tunnel: w653 -> [w668 _]
              tunnel: w652 -> [w664 w687]
              frame "None", Default {
                # "Stays in Task 5_A until stepper reaches desired \nheight"
                # "T: Go back to idle, F: Continue with task\""
                # ">> Manual override >>"
                n249 = case shown="True" w669 {
                  tunnel: [w677 w683] -> w673
                  tunnel: w664 -> [w675 w681]
                  frame False {
                    n250 = for {
                      tunnel: string[] ["Z STEPPER CAM HEIGHT", "READ STEPPER VALUES"] ("element") -> [w678] mode=indexing
                      shift-right: [w680] -> w677
                      shift-left: w675 -> [w679]
                      n251 = Enqueue Element(queue=w679, element=w678) -> (queue out=w680:refnum<queue>)  [unwired: 2 in, 2 out]
                    }
                  }
                  frame True {
                    n252 = for {
                      shift-right: [w685] -> w683
                      shift-left: w681 -> [w686]
                      tunnel: string[] ["OPEN LOG CAM", "SET TIMER", ""] -> [w684] mode=indexing
                      n253 = Enqueue Element(queue=w686, element=w684) -> (queue out=w685:refnum<queue>)  [unwired: 2 in, 2 out]
                    }
                  }
                }
                n254 = Or(x=w669, y=w668) -> (x .or. y?=w671:bool)
                n255 = Select(t=State_Type_Definitions."True Stop" ("Enum"), s=w668, f=State_Type_Definitions."Task 5 _B" ("Enum")) -> (s? t:f=w665:u16)
                n256 = Select(t=w665, s=w671, f=State_Type_Definitions."Task 5_A" ("Enum")) -> (s? t:f=w670:u16)
              }
              frame "Exit" {
                n257 = for {
                  shift-right: [w693] -> w690
                  shift-left: w687 -> [w694]
                  tunnel: string[] ["STOP", "RESET ENCODERS", "RESET YAW", "ARDUINO MODE 0"] -> [w692] mode=indexing
                  n258 = Enqueue Element(queue=w694, element=w692) -> (queue out=w693:refnum<queue>)  [unwired: 2 in, 2 out]
                }
              }
            }
          }
          frame 13 {
            # ">>> yStepper command>>>"
            n259 = Dequeue Element(queue=w698, timeout in ms (-1)=w697, error in (no error)=w699) -> (element=w696:T7)  [unwired: 3 out]
            n260 = And(x=w701, y=w702) -> (x .and. y?=w700:bool)
            "Recognized object + Time up?" <- w700
            n261 = case shown="\"None\", Default" w696 {
              tunnel: [w714 State_Type_Definitions."True Stop" ("Enum")] -> w704
              tunnel: [w717 w734] -> w703
              tunnel: [State_Type_Definitions."Idle" ("Enum") State_Type_Definitions."Shutdown" ("Enum")] -> w705
              tunnel: w700 -> [w713 _]
              tunnel: w707 -> [w712 _]
              tunnel: w706 -> [w708 w731]
              frame "None", Default {
                # "Stays in Task 5_B until time is up and object is detected"
                # "T: Go back to idle, F: Continue with task\""
                # ">> Manual override >>"
                n262 = case shown="True" w713 {
                  tunnel: [w721 w727] -> w717
                  tunnel: w708 -> [w719 w725]
                  frame False {
                    n263 = for {
                      tunnel: string[] ["CAM ACQ", "START TIMER"] ("element") -> [w722] mode=indexing
                      shift-right: [w724] -> w721
                      shift-left: w719 -> [w723]
                      n264 = Enqueue Element(queue=w723, element=w722) -> (queue out=w724:refnum<queue>)  [unwired: 2 in, 2 out]
                    }
                  }
                  frame True {
                    n265 = for {
                      shift-right: [w729] -> w727
                      shift-left: w725 -> [w730]
                      tunnel: string[] ["CAM CLOSE", ""] -> [w728] mode=indexing
                      n266 = Enqueue Element(queue=w730, element=w728) -> (queue out=w729:refnum<queue>)  [unwired: 2 in, 2 out]
                    }
                  }
                }
                n267 = Or(x=w713, y=w712) -> (x .or. y?=w715:bool)
                n268 = Select(t=State_Type_Definitions."True Stop" ("Enum"), s=w712, f=State_Type_Definitions."Task 5_C" ("Enum")) -> (s? t:f=w709:u16)
                n269 = Select(t=w709, s=w715, f=State_Type_Definitions."Task 5 _B" ("Enum")) -> (s? t:f=w714:u16)
              }
              frame "Exit" {
                n270 = for {
                  shift-right: [w737] -> w734
                  shift-left: w731 -> [w738]
                  tunnel: string[] ["STOP", "RESET ENCODERS", "RESET YAW", "ARDUINO MODE 0"] -> [w736] mode=indexing
                  n271 = Enqueue Element(queue=w738, element=w736) -> (queue out=w737:refnum<queue>)  [unwired: 2 in, 2 out]
                }
              }
            }
          }
          frame 14 {
            # ">>> yStepper command>>>"
            # ">> Checks if item is in range >>"
            # ">> Manual override >>"
            n272 = Dequeue Element(queue=w750, timeout in ms (-1)=w749, error in (no error)=w748) -> (element=w747:T7)  [unwired: 3 out]
            n273 = In Range and Coerce(upper limit=290.0, x=w743, lower limit=300.0) -> (In Range?=w740:bool)  [unwired: 1 out]
            n274 = case shown="\"None\", Default" w747 {
              tunnel: [w757 State_Type_Definitions."True Stop" ("Enum")] -> w752
              tunnel: [w760 w777] -> w745
              tunnel: [State_Type_Definitions."Idle" ("Enum") State_Type_Definitions."Shutdown" ("Enum")] -> w744
              tunnel: w740 -> [w756 _]
              tunnel: w746 -> [w755 _]
              tunnel: w751 -> [w754 w774]
              frame "None", Default {
                # ">> Is object in range? >>"
                # "Stays in Task 5_C until time is up and object is detected"
                # ">> Manual override >>"
                n275 = case shown="False" w756 {
                  tunnel: [w764 w770] -> w760
                  tunnel: w754 -> [w762 w768]
                  frame False {
                    n276 = for {
                      tunnel: string[] ["CAM ACQ", "START TIMER"] ("element") -> [w765] mode=indexing
                      shift-right: [w767] -> w764
                      shift-left: w762 -> [w766]
                      n277 = Enqueue Element(queue=w766, element=w765) -> (queue out=w767:refnum<queue>)  [unwired: 2 in, 2 out]
                    }
                  }
                  frame True {
                    n278 = for {
                      shift-right: [w772] -> w770
                      shift-left: w768 -> [w773]
                      tunnel: string[] ["CAM CLOSE", ""] -> [w771] mode=indexing
                      n279 = Enqueue Element(queue=w773, element=w771) -> (queue out=w772:refnum<queue>)  [unwired: 2 in, 2 out]
                    }
                  }
                }
                n280 = Or(x=w756, y=w755) -> (x .or. y?=w758:bool)
                n281 = Select(t=State_Type_Definitions."True Stop" ("Enum"), s=w758, f=State_Type_Definitions."Task 5_C_Error" ("Enum")) -> (s? t:f=w757:u16)
              }
              frame "Exit" {
                n282 = for {
                  shift-right: [w780] -> w777
                  shift-left: w774 -> [w781]
                  tunnel: string[] ["STOP", "RESET ENCODERS", "RESET YAW", "ARDUINO MODE 0"] -> [w779] mode=indexing
                  n283 = Enqueue Element(queue=w781, element=w779) -> (queue out=w780:refnum<queue>)  [unwired: 2 in, 2 out]
                }
              }
            }
          }
          frame 15 {
            # ">>> yStepper command>>>"
            # ">> Checks if yStepper has reached target>>"
            n284 = Dequeue Element(queue=w792, timeout in ms (-1)=w791, error in (no error)=w790) -> (element=w789:T7)  [unwired: 3 out]
            n285 = formula code="if (pos < 170)\ny = 40;\n\nelse if (pos >= 170 && pos <= 320)\ny = 20;\n\nelse if (pos > 320)\ny = 0;"("pos"=w782) -> ("y"=w786:dbl)
            n286 = To Unsigned Byte Integer(number=w786) -> (unsigned 8bit integer=w784:u8)
            n287 = Equal?(x=w785, y=w784) -> (x = y?=w783:bool)
            n288 = case shown="\"None\", Default" w789 {
              tunnel: [w804 State_Type_Definitions."True Stop" ("Enum")] -> w796
              tunnel: [w807 w824] -> w795
              tunnel: [State_Type_Definitions."Idle" ("Enum") State_Type_Definitions."Shutdown" ("Enum")] -> w797
              tunnel: w793 -> [w803 _]
              tunnel: w794 -> [w799 w821]
              tunnel: w783 -> [w798 _]
              frame "None", Default {
                # ">> T: Breaks out of state loop; F: Stays in loop>>"
                # ">> Manual override >>"
                # ">> Checks if yStepper has reached target>>"
                # "Stays in Task 5_C until time is up and object is detected"
                # "T: Go back to idle, F: Continue with task\""
                # ">> Manual override >>"
                n289 = case shown="True" w798 {
                  tunnel: [w811 w817] -> w807
                  tunnel: w799 -> [w809 w815]
                  frame False {
                    n290 = for {
                      tunnel: string[] ["Y STEPPER CONTROL", "READ STEPPER VALUES"] ("element") -> [w812] mode=indexing
                      shift-right: [w814] -> w811
                      shift-left: w809 -> [w813]
                      n291 = Enqueue Element(queue=w813, element=w812) -> (queue out=w814:refnum<queue>)  [unwired: 2 in, 2 out]
                    }
                  }
                  frame True {
                    n292 = for {
                      shift-right: [w819] -> w817
                      shift-left: w815 -> [w820]
                      tunnel: string[] ["OPEN LOG CAM", ""] -> [w818] mode=indexing
                      n293 = Enqueue Element(queue=w820, element=w818) -> (queue out=w819:refnum<queue>)  [unwired: 2 in, 2 out]
                    }
                  }
                }
                n294 = Or(x=w798, y=w803) -> (x .or. y?=w805:bool)
                n295 = Select(t=State_Type_Definitions."True Stop" ("Enum"), s=w803, f=State_Type_Definitions."Task 5 _B" ("Enum")) -> (s? t:f=w800:u16)
                n296 = Select(t=w800, s=w805, f=State_Type_Definitions."Task 5_C_Error" ("Enum")) -> (s? t:f=w804:u16)
              }
              frame "Exit" {
                n297 = for {
                  shift-right: [w827] -> w824
                  shift-left: w821 -> [w828]
                  tunnel: string[] ["STOP", "RESET ENCODERS", "RESET YAW", "ARDUINO MODE 0"] -> [w826] mode=indexing
                  n298 = Enqueue Element(queue=w828, element=w826) -> (queue out=w827:refnum<queue>)  [unwired: 2 in, 2 out]
                }
              }
            }
            n299 = Bundle By Name(cluster=w788, "yStepper desired"=w784) -> (w787:T8)
          }
          frame 23 {
            # ">>> yStepper command>>>"
            n300 = Dequeue Element(queue=w836, timeout in ms (-1)=w835, error in (no error)=w834) -> (element=w841:T7)  [unwired: 3 out]
            n301 = Equal?(x=w832, y=u8 80) -> (x = y?=w831:bool)
            n302 = case shown="\"None\", Default" w841 {
              tunnel: [w848 State_Type_Definitions."True Stop" ("Enum")] -> w839
              tunnel: [w847 w865] -> w838
              tunnel: [State_Type_Definitions."Idle" ("Enum") State_Type_Definitions."Shutdown" ("Enum")] -> w840
              tunnel: w837 -> [w843 _]
              tunnel: w833 -> [w845 _]
              tunnel: w831 -> [w842 _]
              frame "None", Default {
                n303 = case shown="False" w842 {
                  tunnel: [w853 w859] -> w847
                  tunnel: w845 -> [w851 w857]
                  frame False {
                    n304 = for {
                      tunnel: string[] ["Z STEPPER CAM HEIGHT", "READ STEPPER VALUES"] ("element") -> [w854] mode=indexing
                      shift-right: [w856] -> w853
                      shift-left: w851 -> [w855]
                      n305 = Enqueue Element(queue=w855, element=w854) -> (queue out=w856:refnum<queue>)  [unwired: 2 in, 2 out]
                    }
                  }
                  frame True {
                    n306 = for {
                      shift-right: [w861] -> w859
                      shift-left: w857 -> [w862]
                      tunnel: string[] ["CAM ACQ", ""] -> [w860] mode=indexing
                      n307 = Enqueue Element(queue=w862, element=w860) -> (queue out=w861:refnum<queue>)  [unwired: 2 in, 2 out]
                    }
                  }
                }
                n308 = Or(x=w842, y=w843) -> (x .or. y?=w844:bool)
                n309 = Select(t=State_Type_Definitions."Task 6_B" ("Enum"), s=w844, f=State_Type_Definitions."Task 6_A" ("Enum")) -> (s? t:f=w848:T6)
              }
              frame "Exit" {
                n310 = for {
                  shift-right: [w868] -> w865
                  shift-left: _ -> [w869]
                  tunnel: string[] ["STOP", "RESET ENCODERS", "RESET YAW", "ARDUINO MODE 0"] -> [w867] mode=indexing
                  n311 = Enqueue Element(queue=w869, element=w867) -> (queue out=w868:refnum<queue>)  [unwired: 2 in, 2 out]
                }
              }
            }
          }
          frame 24 {
            # ">>> yStepper command>>>"
            n312 = Dequeue Element(queue=w879, timeout in ms (-1)=w877, error in (no error)=w878) -> (element=w876:T7)  [unwired: 3 out]
            n313 = case shown="\"None\", Default" w876 {
              tunnel: [w886 State_Type_Definitions."True Stop" ("Enum")] -> w872
              tunnel: [w885 w904] -> w880
              tunnel: [State_Type_Definitions."Idle" ("Enum") State_Type_Definitions."Shutdown" ("Enum")] -> w873
              tunnel: w875 -> [w881 _]
              tunnel: w874 -> [w883 _]
              tunnel: w871 -> [w882 w901]
              frame "None", Default {
                # ">> Manual override >>"
                n314 = case shown="True" w883 {
                  tunnel: [w891 w897] -> w885
                  tunnel: w882 -> [w890 w895]
                  frame False {
                    n315 = for {
                      shift-right: [w894] -> w891
                      shift-left: w890 -> [w893]
                      tunnel: string[] ["CAM ACQ", "OPEN CLAW"] -> [w892] mode=indexing
                      n316 = Enqueue Element(queue=w893, element=w892) -> (queue out=w894:refnum<queue>)  [unwired: 2 in, 2 out]
                    }
                  }
                  frame True {
                    n317 = for {
                      shift-right: [w899] -> w897
                      shift-left: w895 -> [w900]
                      tunnel: string[] ["CAM ACQ", "CLOSE CLAW"] -> [w898] mode=indexing
                      n318 = Enqueue Element(queue=w900, element=w898) -> (queue out=w899:refnum<queue>)  [unwired: 2 in, 2 out]
                    }
                  }
                }
                n319 = Select(t=State_Type_Definitions."True Stop" ("Enum"), s=w881, f=State_Type_Definitions."Task 6_B" ("Enum")) -> (s? t:f=w886:T6)
              }
              frame "Exit" {
                # ">> State after true stop >>"
                # ">> Goes to true stop >>"
                n320 = for {
                  shift-right: [w907] -> w904
                  shift-left: w901 -> [w908]
                  tunnel: string[] ["STOP", "RESET ENCODERS", "RESET YAW", ""] -> [w906] mode=indexing
                  n321 = Enqueue Element(queue=w908, element=w906) -> (queue out=w907:refnum<queue>)  [unwired: 2 in, 2 out]
                }
              }
            }
          }
        }
      }
    }
  }
  n322 = call <vilib>:"DIO Close.vi"("error in (no error)"=w24, "DIO Info In"=w27) -> ()  [unwired: 9 in, 1 out]
  n323 = call <vilib>:"DIO Close.vi"("error in (no error)"=w34, "DIO Info In"=w36) -> ()  [unwired: 9 in, 1 out]
  n324 = call <vilib>:"NavX Close.vi"("error in (no error)"=w5, "NavX Info In"=w4) -> ()  [unwired: 9 in, 1 out]
  n325 = call <vilib>:"DIO Close.vi"("error in (no error)"=w29, "DIO Info In"=w31) -> ()  [unwired: 9 in, 1 out]
  n326 = call <vilib>:"DIO Close.vi"("error in (no error)"=w12, "DIO Info In"=w13) -> ()  [unwired: 9 in, 1 out]
  n327 = call <vilib>:"DIO Close.vi"("error in (no error)"=w7, "DIO Info In"=w8) -> ()  [unwired: 9 in, 1 out]
  n328 = while {
    stop <- w1315 stop-if-true
    n329 = call <vilib>:"RT Get CPU Loads.vi"() -> ("CPU loads"=→"CPU loads":T5[])  [unwired: 10 in, 1 out]
    n330 = Wait (ms)(milliseconds to wait=u32 100) -> ()  [unwired: 1 out]
    n331 = call "FGV Bool.vi"("Init/Read/Write State"=States_for_Action_Engine."Read") -> ("Output node"=w1315:bool)  [unwired: 2 in, 1 out]
  }
  n332 = Merge Errors "Merge Errors"(w64, w63) -> (w46:errorcluster)
  n333 = Merge Errors(w50, w46) -> (w45:errorcluster)
  n334 = Destroy User Event(user event=w67, error in=w45) -> ()  [unwired: 1 out]
  n335 = Destroy User Event(user event=w68, error in=w45) -> ()  [unwired: 1 out]
  n336 = Unregister For Events(event registration refnum=w59, error in=w45) -> ()  [unwired: 1 out]
  n337 = Release Queue(queue=w41, error in (no error)=w45) -> (error out=w23:errorcluster)  [unwired: 1 in, 2 out]
  n338 = Release Queue(queue=w58, error in (no error)=w45) -> ()  [unwired: 1 in, 3 out]
  n339 = call <vilib>:"Simple Error Handler.vi"("error in (no error)"=w23) -> ("error out"=w22:errorcluster)  [unwired: 4 in, 4 out]
  n340 = call <vilib>:"Reset myRIO.vi"("error in (no error)"=w22) -> ("error out"=→"error out":errorcluster)  [unwired: 10 in]
